vi "Gamepad MicroDrive Control with limits.vi"() -> ()   [LabVIEW 2012]
uses:
  <vilib>/Utility/miscctls.llb/LVPointTypeDef.ctl
  <vilib>/Utility/file.llb/Read From Spreadsheet File (I64).vi
  <vilib>/Utility/inputDevices.llb/closeJoystick.vi
  <vilib>/Utility/inputDevices.llb/joystickAcquire.vi
  <vilib>/Utility/file.llb/Write To Spreadsheet File (DBL).vi
  <vilib>/Utility/file.llb/Read From Spreadsheet File (DBL).vi
  MicroDrive.dll
panel:
  in  "xf":u16(ring)=3 items=["1 X"=1, "2 A"=2, "3 B"=3, "4 Y"=4, "5 LB"=5, "6 RB"=6, "7 LT"=7, "8 RT"=8, "9 Back"=9]
  in  "zf":u16(ring)=6 items=["1 X"=1, "2 A"=2, "3 B"=3, "4 Y"=4, "5 LB"=5, "6 RB"=6, "7 LT"=7, "8 RT"=8, "9 Back"=9]
  in  "Slide 2":cluster{u32, u32, u32}(slide)={0, 1, 5} scale=0.0..7.0
  in  "Invert 2":bool=TRUE
  out "z top":bool
  out "M3 encoder at position":dbl=5.0 step=0.1 format="%_6g"
  in  "M3 low limit":dbl=-10.0 step=0.1 format="%_6g"
  in  "M3 high limit":dbl=10.0 step=0.1 format="%_6g"
  in  "Reset Z":bool
  out "E3 encoder":dbl=5.0 step=0.1 format="%_6g"
  in  "M3 velocity":dbl=1.0 min=0.01905 max=4.0 format="%.3f"
  in  "M3 distance":dbl=1.0 format="%.5f"
  in  "z-down":bool
  in  "z-up":bool
  in  "readWhileMoving":bool=TRUE
  in  "loadLimits":bool
  in  "saveLimits":bool
  in  "roiLoad":bool
  in  "roiSave":bool
  in  "roiRename":bool
  in  "roiName":string
  in  "roiDeleteAll":bool
  out "M2 encoder at position":dbl=5.0 step=0.1 format="%_6g"
  out "M1 encoder at position":dbl=5.0 step=0.1 format="%_6g"
  in  "M2 distance":dbl=1.0 format="%.5f"
  in  "M1 distance":dbl=1.0 format="%.5f"
  out "E2 encoder":dbl=5.0 step=0.1 format="%_6g"
  out "E1 encoder":dbl=5.0 step=0.1 format="%_6g"
  in  "left":bool
  in  "down":bool
  in  "right":bool
  in  "up":bool
  in  "roiMoveTo":bool
  in  "roiDelete":bool
  in  "roiAdd":bool
  in  "ROIs":u16(ring)
  in  "Use software limits":bool=TRUE
  in  "M2 low limit":dbl=-10.0 step=0.1 format="%_6g"
  in  "M2 high limit":dbl=10.0 step=0.1 format="%_6g"
  in  "M1 low limit":dbl=-10.0 step=0.1 format="%_6g"
  in  "M1 high limit":dbl=10.0 step=0.1 format="%_6g"
  in  "closed?":bool
  in  "configure":bool
  in  "device info":bool
  in  "yf":u16(ring)=4 items=["1 X"=1, "2 A"=2, "3 B"=3, "4 Y"=4, "5 LB"=5, "6 RB"=6, "7 LT"=7, "8 RT"=8, "9 Back"=9]
  in  "halt 3":u16(ring)=9 items=["1 X"=1, "2 A"=2, "3 B"=3, "4 Y"=4, "5 LB"=5, "6 RB"=6, "7 LT"=7, "8 RT"=8, "9 Back"=9]
  in  "yr":u16(ring)=2 items=["1 X"=1, "2 A"=2, "3 B"=3, "4 Y"=4, "5 LB"=5, "6 RB"=6, "7 LT"=7, "8 RT"=8, "9 Back"=9]
  in  "zr":u16(ring)=8 items=["1 X"=1, "2 A"=2, "3 B"=3, "4 Y"=4, "5 LB"=5, "6 RB"=6, "7 LT"=7, "8 RT"=8, "9 Back"=9]
  in  "xr":u16(ring)=1 items=["1 X"=1, "2 A"=2, "3 B"=3, "4 Y"=4, "5 LB"=5, "6 RB"=6, "7 LT"=7, "8 RT"=8, "9 Back"=9]
  out "right":bool
  out "left":bool
  out "top":bool
  in  "halt 2":bool
  out "bottom":bool
  out "Max Velocity One Axis":dbl
  out "Min Velocity":dbl
  in  "Reset Both":bool
  in  "Reset Y":bool
  in  "Reset X":bool
  in  "M2 velocity":dbl=1.0 min=0.01905 max=4.0 format="%.3f"
  in  "M1 velocity":dbl=1.0 min=0.01905 max=4.0 format="%.3f"
  out "Max VelocityTwo Axis":dbl format="%.3f"
  in  "Invert":bool=TRUE
  in  "Invert":bool
  out "z bottom":bool
  # "Current Postion"
  # "Single Step Controls"
  # "Stage-Position List"
  # "Encoders"
  # "Step distance"
  # "mm"
  # "mm"
  # "mm"
  # "mm"
  # "mm"
  # "mm"
  # "mm"
  # "mm"
  # "Step velocity"
  # "mm"
  # "mm"
  # "mm"
  # "Read encoders while moving"
  # "Disable if MicroDrive exhibits irregularities while moving."
  # "mm/s"
  # "mm/s"
  # "Rename"
  # "Reset Encoders"
  # "mm/s"
  # "Step Velocity also sets maximum velocity  achievable with gamepad."
  # "Add/Remove"
  # "Reseting encoders will alter Software Limits and erase ROIs"
  # "Software Limits"
  # "(mm)"
  # "Software limits are based on encoder values as displayed above. CAUTION: stage may stop up to 0.5mm beyond specified limit."
  # "Configuration"
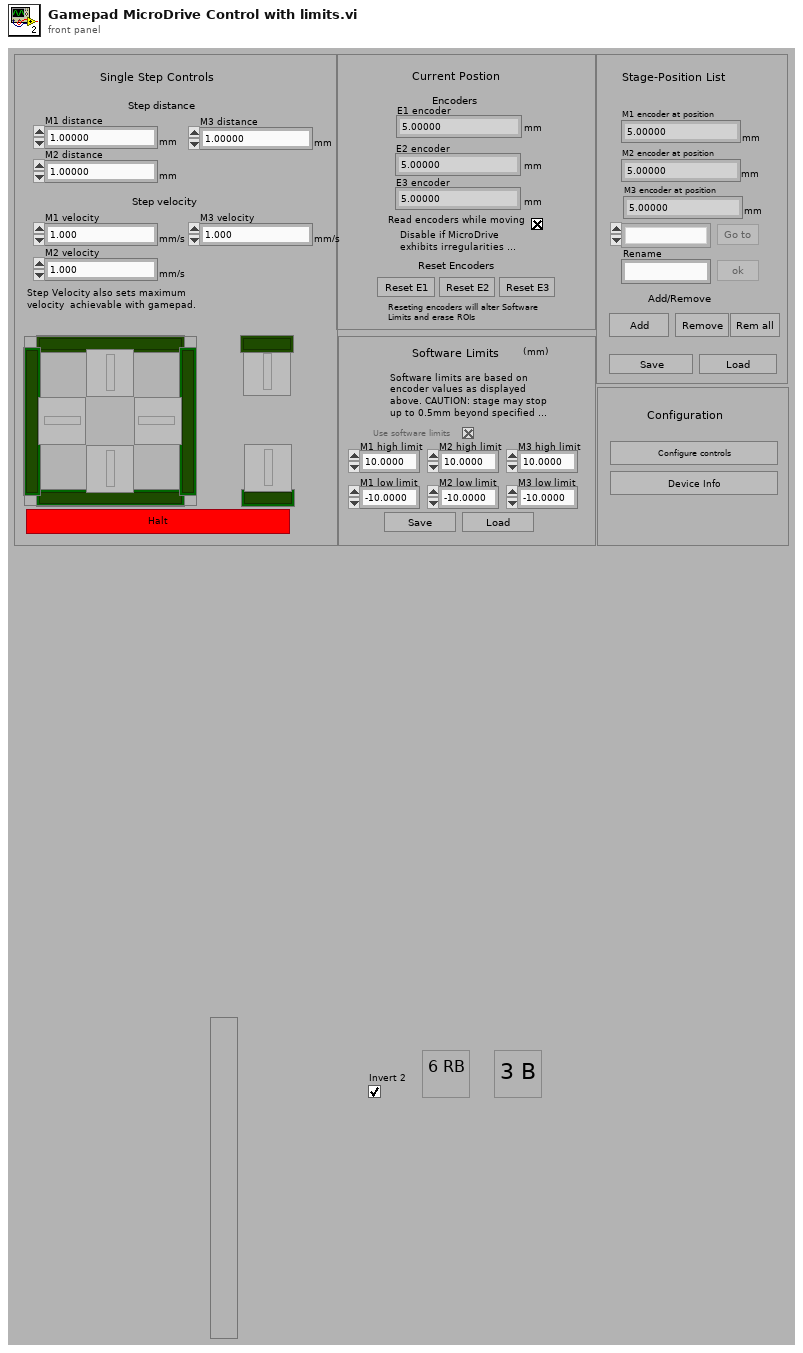
[diagram p1: front panel]
types:
  T1 = enum16{"open", "replace", "create", "open or create", "replace or create", "replace or create with confirmation"}
  T2 = typedef "LVPointTypeDef.ctl" = cluster{"Horizontal":i16, "Vertical":i16}
  T3 = enum8{"Enabled", "Disabled", "Disabled and Grayed Out"}
  T4 = cluster{"Controls":cluster{"Values":cluster{"up":u16, "right":u16}}, "ControlRefs":cluster{"Values":cluster{"up":refnum<vi>, "right":refnum<vi>}}, "Variables":cluster{"Commands":cluster{"up_changed":bool, "right_changed":bool}}}
  T5 = cluster{"Controls":cluster{"Commands":cluster{"right":bool, "left":bool, "up":bool, "down":bool, "z-up":bool, "z-down":bool}, "Values":cluster{"xStep":dbl, "yStep":dbl, "xVelocity":dbl, "yVelocity":dbl, "zStep":dbl, "zVelocity":dbl}}, "ControlRefs":cluster{"Commands":cluster{"right":refnum<vi>, "left":refnum<vi>, "up":refnum<vi>, "down":refnum<vi>, "z-up":refnum<vi>, "z-down":refnum<vi>}, "Values":cluster{"X step":refnum<vi>, "Y step":refnum<vi>, "xVelocity":refnum<vi>, "yVelocity":refnum<vi>, "Z step":refnum<vi>, "zVelocity":refnum<vi>}}}
  T6 = cluster{"Controls":cluster{"Commands":cluster{"Use software limits":bool, "reset X":bool, "reset Y":bool, "reset All":bool, "saveLimits":bool, "loadLimits":bool, "Read encoders while moving":bool, "reset Z":bool}, "Values":cluster{"X high limit":dbl, "X low limit":dbl, "Y high limit":dbl, "Y low limit":dbl, "xEnc":dbl, "yEnc":dbl, "Z high limit":dbl, "Z low limit":dbl, "zEnc":dbl}}, "ControlRefs":cluster{"Commands":cluster{"Use software limits":refnum<vi>, "reset X":refnum<vi>, "reset Y":refnum<vi>, "reset All":refnum<vi>, "saveLimits":refnum<vi>, "loadLimits":refnum<vi>, "Read encoders while moving":refnum<vi>, "reset Z":refnum<vi>}, "Values":cluster{"X high limit":refnum<vi>, "X low limit":refnum<vi>, "Y high limit":refnum<vi>, "Y low limit":refnum<vi>, "xEnc":refnum<vi>, "yEnc":refnum<vi>, "Z high limit":refnum<vi>, "Z low limit":refnum<vi>, "zEnc":refnum<vi>}}, "Variables":cluster{"Commands":cluster{"softLimit_xHigh":bool, "softLimit_xLow":bool, "softLimit_yHigh":bool, "softLimit_yLow":bool, "softLimit_zHigh":bool, "softLimit_zLow ":bool}}}
  T7 = cluster{"Controls":cluster{"Commands":cluster{"roiMoveTo":bool, "roiAdd":bool, "roiDelete":bool, "roiDeleteAll":bool, "rename":bool, "roiSave":bool, "roiLoad":bool}, "Values":cluster{"ROIs":u16, "roiName":string}}, "ControlRefs":cluster{"Commands":cluster{"roiMoveTo":refnum<vi>, "roiAdd":refnum<vi>, "roiDelete":refnum<vi>, "roiDeleteAll":refnum<vi>, "rename":refnum<vi>, "roiSave":refnum<vi>, "roiLoad":refnum<vi>}, "Values":cluster{"ROIs":refnum<vi>, "roiName":refnum<vi>}}, "Variables":cluster{"Values":cluster{"roiText":string[], "ROIs":cluster{"x":dbl, "y":dbl, "z":dbl}[], "roiNumItems":i32}}}
  T8 = cluster{"xr":refnum<vi>, "yr":refnum<vi>, "xf":refnum<vi>, "yf":refnum<vi>, "zr":refnum<vi>, "zf":refnum<vi>, "halt 3":refnum<vi>}
  T9 = cluster{"X axis":i32, "Y axis":i32, "Z axis":i32, "X axis rotation":i32, "Y axis rotation":i32, "Z axis rotation":i32, "U axis":i32, "V axis":i32}
  T10 = cluster{"button 1":bool, "button 2":bool, "button 3":bool, "button 4":bool, "button 5":bool, "button 6":bool, "button 7":bool, "button 8":bool, "button 9":bool, "button 10":bool, "button 11":bool, "button 12":bool, "button 13":bool, "button 14":bool, "button 15":bool, "button 16":bool, "button 17":bool, "button 18":bool, "button 19":bool, "button 20":bool, "button 21":bool, "button 22":bool, "button 23":bool, "button 24":bool, "button 25":bool, "button 26":bool, "button 27":bool, "button 28":bool, "button 29":bool, "button 30":bool, "button 31":bool, "button 32":bool}
  T11 = cluster{"left":bool, "down":bool, "right":bool, "up":bool, "z-up":bool, "z-down":bool, "halt":bool, "button 10":bool}
  T12 = cluster{"y reverse":bool, "y foward":bool, "x reverse":bool, "x foward":bool, "z reverse":bool, "z foward":bool}
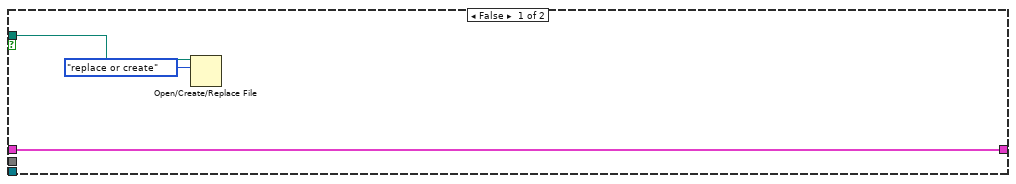
[diagram p2: hidden frame]
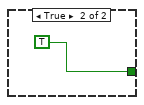
[diagram p4: hidden frame]
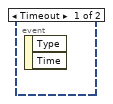
[diagram p8: hidden frame]
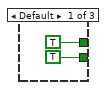
[diagram p13: hidden frame]
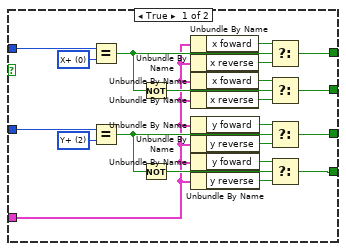
[diagram p15: hidden frame]
diagram:
  n1 = flat-sequence {
    tunnel: [w65] -> w22
    tunnel: [w64] -> w24
    tunnel: [w63] -> w26
    tunnel: [w62] -> w20
    tunnel: [w61] -> w18
    tunnel: w26 -> [w84]
    tunnel: [w84] -> w25
    tunnel: w24 -> [w83]
    tunnel: [w83] -> w23
    tunnel: w22 -> [w82]
    tunnel: [w82] -> w21
    tunnel: w20 -> [w77]
    tunnel: [w75] -> w19
    tunnel: w18 -> [w70]
    tunnel: [w70] -> w17
    tunnel: [w85] -> w10
    tunnel: [w100] -> w8
    tunnel: [w87] -> w6
    tunnel: [w86] -> w4
    tunnel: [w99] -> w2
    tunnel: w17 -> [w99]
    tunnel: w19 -> [w86]
    tunnel: w21 -> [w85]
    tunnel: w23 -> [w95]
    tunnel: w25 -> [w87]
    tunnel: w10 -> [w124]
    tunnel: [w124] -> w9
    tunnel: w8 -> [w123]
    tunnel: [w123] -> w7
    tunnel: w6 -> [w107]
    tunnel: [w106] -> w5
    tunnel: w4 -> [w122]
    tunnel: [w122] -> w3
    tunnel: w2 -> [w121]
    tunnel: [w121] -> w1
    tunnel: w9 -> [w131]
    tunnel: [w125] -> w30
    tunnel: w7 -> [w137]
    tunnel: [w137] -> w29
    tunnel: w5 -> [w136]
    tunnel: [w136] -> w28
    tunnel: w3 -> [w135]
    tunnel: [w135] -> w27
    tunnel: w1 -> [w130]
    tunnel: [w130] -> w16
    tunnel: w30 -> [w145]
    tunnel: [w145] -> w34
    tunnel: w29 -> [w142]
    tunnel: [w142] -> w33
    tunnel: w28 -> [w151]
    tunnel: [w151] -> w32
    tunnel: w27 -> [w150]
    tunnel: [w150] -> w31
    tunnel: w16 -> [w141]
    tunnel: [w140] -> w13
    tunnel: [w204] -> w50
    tunnel: [w207] -> w45
    tunnel: [w206] -> w44
    tunnel: [w205] -> w37
    tunnel: w31 -> [w205]
    tunnel: w32 -> [w206]
    tunnel: w33 -> [w207]
    tunnel: w34 -> [w204]
    tunnel: [w194] -> w14
    tunnel: w13 -> [w194]
    tunnel: [w214] -> w54
    tunnel: [w213] -> w53
    tunnel: w50 -> [w212]
    tunnel: [w212] -> w49
    tunnel: [w211] -> w46
    tunnel: w45 -> [w211]
    tunnel: w44 -> [w210]
    tunnel: [w210] -> w42
    tunnel: [w209] -> w38
    tunnel: w37 -> [w209]
    tunnel: [w208] -> w15
    tunnel: w14 -> [w208]
    tunnel: [w243] -> w60
    tunnel: [w244] -> w58
    tunnel: [w240] -> w56
    tunnel: w54 -> [w244]
    tunnel: w53 -> [w243]
    tunnel: w49 -> [w239]
    tunnel: [w239] -> w47
    tunnel: w46 -> [w237]
    tunnel: [w238] -> w43
    tunnel: w42 -> [w238]
    tunnel: [w237] -> w41
    tunnel: w38 -> [w236]
    tunnel: [w236] -> w35
    tunnel: w15 -> [w235]
    tunnel: [w235] -> w11
    tunnel: w60 -> [w270]
    tunnel: [w270] -> w59
    tunnel: w58 -> [w271]
    tunnel: [w271] -> w57
    tunnel: w56 -> [w269]
    tunnel: [w269] -> w55
    tunnel: [w264] -> w52
    tunnel: [u32 0 ("current button state")] -> w51
    tunnel: [w262] -> w48
    tunnel: w47 -> [w262]
    tunnel: w43 -> [w260]
    tunnel: w41 -> [w261]
    tunnel: [w261] -> w40
    tunnel: [w260] -> w39
    tunnel: [w259] -> w36
    tunnel: w35 -> [w259]
    tunnel: [w258] -> w12
    tunnel: w11 -> [w258]
    tunnel: w55 -> [w279]
    tunnel: w57 -> [w281]
    tunnel: w59 -> [w280]
    tunnel: w52 -> [w278]
    tunnel: w51 -> [w277]
    tunnel: w48 -> [w276]
    tunnel: w40 -> [w275]
    tunnel: w39 -> [w274]
    tunnel: w36 -> [w273]
    tunnel: w12 -> [w272]
    frame #0 {
      w61 = T4 {"Controls"={"Values"={"up"=2, "right"=0}}, "ControlRefs"={"Values"={"up"=refnum, "right"=refnum}}, "Variables"={"Commands"={"up_changed"=FALSE, "right_changed"=FALSE}}}  # Configuration
      w62 = T5 {"Controls"={"Commands"={"right"=FALSE, "left"=FALSE, "up"=FALSE, "down"=FALSE, "z-up"=FALSE, "z-down"=FALSE}, "Values"={"xStep"=1.0, "yStep"=1.0, "xVelocity"=1.0, "yVelocity"=1.0, "zStep"=1.0, "zVelocity"=1.0}}, "ControlRefs"={"Commands"={"right"=refnum, "left"=refnum, "up"=refnum, "down"=refnum, "z-up"=refnum, "z-down"=refnum}, "Values"={"X step"=refnum, "Y step"=refnum, "xVelocity"=refnum, "yVelocity"=refnum, "Z step"=refnum, "zVelocity"=refnum}}}  # Motion
      w63 = T6 {"Controls"={"Commands"={"Use software limits"=FALSE, "reset X"=FALSE, "reset Y"=FALSE, "reset All"=FALSE, "saveLimits"=FALSE, "loadLimits"=FALSE, "Read encoders while moving"=FALSE, "reset Z"=FALSE}, "Values"={"X high limit"=100.0, "X low limit"=-100.0, "Y high limit"=100.0, "Y low limit"=-100.0, "xEnc"=0.0, "yEnc"=0.0, "Z high limit"=100.0, "Z low limit"=-100.0, "zEnc"=0.0}}, "ControlRefs"={"Commands"={"Use software limits"=refnum, "reset X"=refnum, "reset Y"=refnum, "reset All"=refnum, "saveLimits"=refnum, "loadLimits"=refnum, "Read encoders while moving"=refnum, "reset Z"=refnum}, "Values"={"X high limit"=refnum, "X low limit"=refnum, "Y high limit"=refnum, "Y low limit"=refnum, "xEnc"=refnum, "yEnc"=refnum, "Z high limit"=refnum, "Z low limit"=refnum, "zEnc"=refnum}}, "Variables"={"Commands"={"softLimit_xHigh"=FALSE, "softLimit_xLow"=FALSE, "softLimit_yHigh"=FALSE, "softLimit_yLow"=FALSE, "softLimit_zHigh"=FALSE, "softLimit_zLow "=FALSE}}}  # Encoder
      w64 = T7 {"Controls"={"Commands"={"roiMoveTo"=FALSE, "roiAdd"=FALSE, "roiDelete"=FALSE, "roiDeleteAll"=FALSE, "rename"=FALSE, "roiSave"=FALSE, "roiLoad"=FALSE}, "Values"={"ROIs"=0, "roiName"=""}}, "ControlRefs"={"Commands"={"roiMoveTo"=refnum, "roiAdd"=refnum, "roiDelete"=refnum, "roiDeleteAll"=refnum, "rename"=refnum, "roiSave"=refnum, "roiLoad"=refnum}, "Values"={"ROIs"=refnum, "roiName"=refnum}}, "Variables"={"Values"={"roiText"=[], "ROIs"=[], "roiNumItems"=0}}}  # ROIs
      w65 = T8 {"xr"=refnum, "yr"=refnum, "xf"=refnum, "yf"=refnum, "zr"=refnum, "zf"=refnum, "halt 3"=refnum}  # output cluster
    }
    frame #1 {
      n2 = control-ref of="right"() -> (w74:refnum<vi>)
      n3 = control-ref of="left"() -> (w73:refnum<vi>)
      n4 = control-ref of="up"() -> (w72:refnum<vi>)
      n5 = control-ref of="down"() -> (w71:refnum<vi>)
      n6 = control-ref of="z-up"() -> (w69:refnum<vi>)
      n7 = control-ref of="z-down"() -> (w68:refnum<vi>)
      n8 = control-ref of="M1 distance"() -> (w78:refnum<vi>)
      n9 = control-ref of="M2 distance"() -> (w79:refnum<vi>)
      n10 = control-ref of="M1 velocity"() -> (w80:refnum<vi>)
      n11 = control-ref of="M2 velocity"() -> (w81:refnum<vi>)
      n12 = control-ref of="M3 distance"() -> (w67:refnum<vi>)
      n13 = control-ref of="M3 velocity"() -> (w66:refnum<vi>)
      n14 = Bundle By Name(cluster=w77, "ControlRefs.Values.X step"=w78, "ControlRefs.Values.Y step"=w79, "ControlRefs.Values.xVelocity"=w80, "ControlRefs.Values.yVelocity"=w81, "ControlRefs.Values.Z step"=w67, "ControlRefs.Values.zVelocity"=w66) -> (w76:T5)
      n15 = Bundle By Name(cluster=w76, "ControlRefs.Commands.right"=w74, "ControlRefs.Commands.left"=w73, "ControlRefs.Commands.up"=w72, "ControlRefs.Commands.down"=w71, "ControlRefs.Commands.z-up"=w69, "ControlRefs.Commands.z-down"=w68) -> (w75:T5)
    }
    frame #2 {
      n16 = control-ref of="roiName"() -> (w90:refnum<vi>)
      n17 = control-ref of="roiMoveTo"() -> (w98:refnum<vi>)
      n18 = control-ref of="roiAdd"() -> (w97:refnum<vi>)
      n19 = control-ref of="roiDelete"() -> (w96:refnum<vi>)
      n20 = control-ref of="roiDeleteAll"() -> (w92:refnum<vi>)
      n21 = control-ref of="roiRename"() -> (w91:refnum<vi>)
      n22 = control-ref of="roiSave"() -> (w89:refnum<vi>)
      n23 = control-ref of="roiLoad"() -> (w88:refnum<vi>)
      n24 = control-ref of="ROIs"() -> (w93:refnum<vi>)
      n25 = Bundle By Name(cluster=w95, "ControlRefs.Values.ROIs"=w93, "ControlRefs.Values.roiName"=w90) -> (w94:T7)
      n26 = Bundle By Name(cluster=w94, "ControlRefs.Commands.roiMoveTo"=w98, "ControlRefs.Commands.roiAdd"=w97, "ControlRefs.Commands.roiDelete"=w96, "ControlRefs.Commands.roiDeleteAll"=w92, "ControlRefs.Commands.rename"=w91, "ControlRefs.Commands.roiSave"=w89, "ControlRefs.Commands.roiLoad"=w88) -> (w100:T7)
    }
    frame #3 {
      n27 = control-ref of="Use software limits"() -> (w108:refnum<vi>)
      n28 = control-ref of="Reset X"() -> (w114:refnum<vi>)
      n29 = control-ref of="Reset Y"() -> (w115:refnum<vi>)
      n30 = control-ref of="Reset Both"() -> (w116:refnum<vi>)
      n31 = control-ref of="saveLimits"() -> (w119:refnum<vi>)
      n32 = control-ref of="loadLimits"() -> (w120:refnum<vi>)
      n33 = control-ref of="readWhileMoving"() -> (w105:refnum<vi>)
      n34 = control-ref of="Reset Z"() -> (w104:refnum<vi>)
      n35 = Bundle By Name(cluster=w107, "ControlRefs.Commands.Use software limits"=w108, "ControlRefs.Commands.reset X"=w114, "ControlRefs.Commands.reset Y"=w115, "ControlRefs.Commands.reset All"=w116, "ControlRefs.Commands.saveLimits"=w119, "ControlRefs.Commands.loadLimits"=w120, "ControlRefs.Commands.Read encoders while moving"=w105, "ControlRefs.Commands.reset Z"=w104) -> (w113:T6)
      n36 = control-ref of="M1 high limit"() -> (w109:refnum<vi>)
      n37 = control-ref of="M1 low limit"() -> (w110:refnum<vi>)
      n38 = control-ref of="M2 high limit"() -> (w111:refnum<vi>)
      n39 = control-ref of="M2 low limit"() -> (w112:refnum<vi>)
      n40 = control-ref of="E1 encoder"() -> (w117:refnum<vi>)
      n41 = control-ref of="E2 encoder"() -> (w118:refnum<vi>)
      n42 = control-ref of="M3 high limit"() -> (w102:refnum<vi>)
      n43 = control-ref of="M3 low limit"() -> (w101:refnum<vi>)
      n44 = control-ref of="E3 encoder"() -> (w103:refnum<vi>)
      n45 = Bundle By Name(cluster=w113, "ControlRefs.Values.X high limit"=w109, "ControlRefs.Values.X low limit"=w110, "ControlRefs.Values.Y high limit"=w111, "ControlRefs.Values.Y low limit"=w112, "ControlRefs.Values.xEnc"=w117, "ControlRefs.Values.yEnc"=w118, "ControlRefs.Values.Z high limit"=w102, "ControlRefs.Values.Z low limit"=w101, "ControlRefs.Values.zEnc"=w103) -> (w106:T6)
    }
    frame #4 {
      n46 = control-ref of="zr"() -> (w126:refnum<vi>)
      n47 = control-ref of="halt 3"() -> (w129:refnum<vi>)
      n48 = control-ref of="xf"() -> (w128:refnum<vi>)
      n49 = control-ref of="zf"() -> (w127:refnum<vi>)
      n50 = control-ref of="xr"() -> (w134:refnum<vi>)
      n51 = control-ref of="yr"() -> (w133:refnum<vi>)
      n52 = control-ref of="yf"() -> (w132:refnum<vi>)
      n53 = Bundle(cluster=w131, "xr"=w134, "yr"=w133, "xf"=w128, "yf"=w132, "zr"=w127, "zf"=w126, "halt 3"=w129) -> (w125:T8)
    }
    frame #5 {
      n54 = control-ref of="This Application"() -> (w149:refnum<vi>)
      n55 = property class="App"(reference=w149) -> ("App.Dir"=w144:path)  [unwired: 1 in, 2 out]
      n56 = control-ref of="Slide 2"() -> (w138:refnum<vi>)
      n57 = Build Path(base path=w144, name or relative path="config.txt") -> (appended path=w147:path)
      n58 = Cluster To Array(cluster=w145) -> (array=w146:refnum<vi>[])
      n59 = call <vilib>:"Check if File or Folder Exists.vi"("path"=w147) -> ("file or folder exists?"=w139:bool, "dup path"=w143:path)  [unwired: 1 in, 8 out]
      n60 = case shown="True" w139 {
        tunnel: w138 -> [_ w168]
        tunnel: w146 -> [_ w167]
        tunnel: w143 -> [w154 w166]
        tunnel: w141 -> [w152 w156]
        tunnel: [w152 w155] -> w140
        frame False {
          n61 = Open/Create/Replace File(file path (use dialog)=w154, operation (0:open)=T1."replace or create") -> ()  [unwired: 1 in, 6 out]
        }
        frame True {
          n62 = Read from Text File(file (use dialog)=w166) -> (text=w165:string)  [unwired: 1 in, 5 out]
          n63 = String To Path(string=w165) -> (path=w164:path)
          n64 = call <vilib>:"Check if File or Folder Exists.vi"("path"=w164) -> ("file or folder exists?"=w162:bool, "dup path"=w158:path)  [unwired: 1 in, 8 out]
          n65 = Not A Number/Path/Refnum?(number/path/refnum=w158) -> (NaN/Path/Refnum?=w161:bool)
          n66 = Empty String/Path?(string/path=w158) -> (empty?=w159:bool)
          n67 = Not(x=w161) -> (.not. x?=w160:bool)
          n68 = Not(x=w159) -> (.not. x?=w157:bool)
          n69 = Compound Arithmetic op=AND(w160, w162, w157) -> (w163:bool)
          n70 = case shown="True" w163 {
            tunnel: w167 -> [_ w188]
            tunnel: w168 -> [_ w189]
            tunnel: w158 -> [_ w187]
            tunnel: w156 -> [w169 w186]
            tunnel: [w169 w185] -> w155
            frame False {
            }
            frame True {
              n71 = call-poly <vilib>:"Read From Spreadsheet File.vi"("transpose (no:F)"=TRUE ("transpose? (no:F)"), "file path (dialog if empty)"=w187) -> ("first row"=w190:i64[])  [unwired: 2 in, 7 out]
              n72 = Array Size(array=w188) -> (size(s)=w184:i32)
              n73 = Split 1D Array(array=w190, index=w184) -> (first subarray=w181:i64[], second subarray=w183:i64[])
              n74 = Index Array(array=w183) -> (element #1=w175:i64, element #2=w176:i64, element #3=w170:i64, element #4=w171:i64, element #5=w172:i64, element #6=w173:i64, element #7=w174:i64)  [unwired: 7 in]
              n75 = Bundle(w176, w175, w170) -> (w182:cluster{i64, i64, i64})  [unwired: 1 out]
              n76 = property class="Slide (strict)"(reference=w189, "Value"=w182) -> ()  [unwired: 1 in, 2 out]
              n77 = Bundle By Name(cluster=w186, "Controls.Values.up"=w173, "Controls.Values.right"=w174) -> (w185:T4)
              n78 = control-ref of="Invert"() -> (w178:refnum<vi>)
              n79 = control-ref of="Invert"() -> (w177:refnum<vi>)
              n80 = Greater Than 0?(x=w171) -> (x > 0?=w180:bool)
              n81 = Greater Than 0?(x=w172) -> (x > 0?=w179:bool)
              n82 = property class="Bool (strict)"(reference=w178, "Value"=w180) -> ()  [unwired: 1 in, 2 out]
              n83 = property class="Bool (strict)"(reference=w177, "Value"=w179) -> ()  [unwired: 1 in, 2 out]
              n84 = for {
                tunnel: w188 -> [w193] mode=indexing
                tunnel: w181 -> [w192] mode=indexing
                n85 = property class="Ring (strict)"(reference=w193, "Value"=w192) -> ()  [unwired: 1 in, 2 out]
              }
            }
          }
        }
      }
    }
    frame #6 {
      w195 = u16 0  # Value
      w196 = string[] []  # Strings
      w200 = TRUE ("Front Panel Window:Closeable")
      w201 = FALSE ("Front Panel Window:Title Bar Visible")
      n86 = Unbundle By Name(w207) -> ("ControlRefs.Values.ROIs"=w197:refnum<vi>)
      n87 = control-ref of="This VI"() -> (w203:refnum<vi>)
      n88 = control-ref of="Pane"() -> (w198:refnum<vi>)
      n89 = property class="Ring (strict)"(reference=w197, "Strings []"=w196, "Value"=w195) -> ()  [unwired: 1 in, 2 out]
      n90 = property class="VI"(reference=w203, "Front Panel.Title"="MicroDrive Gamepad" ("Front Panel Window:Title"), "Front Panel.TitleBarVis"=w200, "TB.Visible"=w201, "Front Panel.ShowMenuBar"=w201, "Front Panel.Closeable"=w200) -> ()  [unwired: 1 in, 2 out]
      n91 = property class="Pane"(reference=w198, "Origin"=T2 {"Horizontal"=0, "Vertical"=0}) -> ()  [unwired: 1 in, 2 out]
    }
    frame #7 {
      n92 = while {
        tunnel: [w220] -> w213
        tunnel: [w215] -> w214
        stop <- w219 stop-if-true
        n93 = flat-sequence {
          tunnel: [w223] -> w222
          tunnel: [w224] -> w221
          tunnel: [w223] -> w218
          tunnel: w222 -> [w228]
          tunnel: [w227] -> w220
          tunnel: w221 -> [w227]
          tunnel: [w226] -> w215
          tunnel: w218 -> [w226]
          tunnel: [w225] -> w217
          frame #0 {
            n94 = call "init joystick.vi"() -> ("device ID"=w224:refnum<k1>, "Joystick found"=w223:bool)  [unwired: 2 out]
          }
          frame #1 {
            n95 = case shown="False" w228 {
              tunnel: [w229 TRUE ("T button?")] -> w225
              frame False {
                n96 = Two Button Dialog(message="Press start (button 10)\n on your Gamepad \n(while pressing 'Ok')\nfor it to be initialized. ", 1:"Cancel Program" ("F button name (\"Cancel\")"), 2:"Ok" ("T button name (\"OK\")")) -> (T button?=w229:bool)
              }
              frame True {
              }
            }
          }
        }
        n97 = Not(x=w217) -> (.not. x?=w216:bool)
        n98 = Or(x=w216, y=w215) -> (x .or. y?=w219:bool)
      }
    }
    frame #8 {
      n99 = dll-call lib="C:/Users/Labview/Desktop/SRR/MicroDrive_x64/Labview Examples/MicroDrive.dll" fn="MCL_InitHandleOrGetExisting"() -> ("return type"=w241:i32)  [unwired: 3 in, 2 out]
      n100 = Less Or Equal To 0?(x=w241) -> (x <= 0?=w242:bool)
      n101 = case shown="True" w242 {
        tunnel: w241 -> [w245 w248]
        tunnel: [w245 w247] -> w240
        tunnel: "Retry" ("T button name (\"OK\")") -> [_ w246]
        frame False {
        }
        frame True {
          n102 = while {
            tunnel: w248 -> [w254]
            tunnel: [w252] -> w247
            tunnel: w246 -> [w249]
            stop <- w251 continue-if-true
            n103 = Two Button Dialog(message="Failed to load MicroDrive!\nRetry?", 2:w249) -> (T button?=w250:bool)  [unwired: 1 out]
            n104 = case shown="True" w250 {
              tunnel: w254 -> [w256 _]
              tunnel: [w256 w257] -> w252
              frame False {
              }
              frame True {
                n105 = dll-call lib="C:/Users/Labview/Desktop/SRR/MicroDrive_x64/Labview Examples/MicroDrive.dll" fn="MCL_InitHandleOrGetExisting"() -> ("return type"=w257:i32)  [unwired: 3 in, 2 out]
              }
            }
            n106 = Less Or Equal To 0?(x=w252) -> (x <= 0?=w253:bool)
            n107 = And(x=w250, y=w253) -> (x .and. y?=w251:bool)
          }
        }
      }
    }
    frame #9 {
      n108 = call "device in.vi"("handle"=w269) -> ("Out"=w264:string, "minVelocity"=→"Min Velocity":dbl, "maxVelocityTwoAxis"=→"Max VelocityTwo Axis":dbl, "maxVelocity"=→"Max Velocity One Axis":dbl)  [unwired: 15 out]
      n109 = local write "closed?"(FALSE ("closed?")) -> ()
    }
    frame #10 {
      n110 = case shown="True" w281 {
        tunnel: w280 -> [_ w293]
        tunnel: w279 -> [_ w290]
        tunnel: w278 -> [_ w289]
        tunnel: w277 -> [_ w287]
        tunnel: w276 -> [_ w286]
        tunnel: w275 -> [_ w285]
        tunnel: w274 -> [_ w284]
        tunnel: w273 -> [_ w283]
        tunnel: w272 -> [_ w282]
        frame False {
        }
        frame True {
          n111 = while {
            tunnel: w293 -> [w537]
            tunnel: [w536] -> w292
            tunnel: [w535] -> w291
            tunnel: w290 -> [w534]
            shift-right: [w527] -> _
            shift-left: w287 -> [w526]
            tunnel: w289 -> [w525]
            tunnel: w286 -> [w517]
            shift-right: [w479] -> _
            shift-left: w285 -> [w495]
            shift-right: [w478] -> _
            shift-left: w284 -> [w494]
            tunnel: w283 -> [w477]
            shift-right: [w401] -> _
            shift-left: w282 -> [w417]
            stop <- w524 stop-if-true
            n112 = flat-sequence {
              tunnel: w477 -> [w546]
              tunnel: w494 -> [w547]
              tunnel: w495 -> [w548]
              tunnel: w517 -> [w549]
              tunnel: w537 -> [w550]
              tunnel: w534 -> [w551]
              tunnel: w526 -> [w552]
              tunnel: w525 -> [w553]
              tunnel: [w553] -> w425
              tunnel: [w552] -> w424
              tunnel: [w551] -> w423
              tunnel: [w550] -> w422
              tunnel: [w549] -> w421
              tunnel: [w548] -> w420
              tunnel: [w547] -> w419
              tunnel: [w545] -> w418
              tunnel: w417 -> [w540]
              tunnel: [w540] -> w416
              tunnel: [w577] -> w382
              tunnel: [w576] -> w380
              tunnel: [w575] -> w378
              tunnel: [w574] -> w376
              tunnel: [w573] -> w374
              tunnel: [w572] -> w372
              tunnel: [w559] -> w370
              tunnel: [w571] -> w368
              tunnel: [w570] -> w366
              tunnel: w416 -> [w570]
              tunnel: w418 -> [w563]
              tunnel: w419 -> [w559]
              tunnel: w420 -> [w566]
              tunnel: w421 -> [w573]
              tunnel: w422 -> [w574]
              tunnel: w423 -> [w575]
              tunnel: w424 -> [w576]
              tunnel: w425 -> [w577]
              tunnel: w382 -> [w602]
              tunnel: [w602] -> w381
              tunnel: w380 -> [w601]
              tunnel: [w601] -> w379
              tunnel: w378 -> [w600]
              tunnel: [w600] -> w377
              tunnel: w376 -> [w599]
              tunnel: [w599] -> w375
              tunnel: w374 -> [w598]
              tunnel: [w598] -> w373
              tunnel: w372 -> [w597]
              tunnel: [w597] -> w371
              tunnel: w370 -> [w585]
              tunnel: [w584] -> w369
              tunnel: w368 -> [w596]
              tunnel: [w596] -> w367
              tunnel: w366 -> [w595]
              tunnel: [w595] -> w365
              tunnel: w381 -> [w615]
              tunnel: [w615] -> w315
              tunnel: w379 -> [w614]
              tunnel: [w614] -> w313
              tunnel: w377 -> [w613]
              tunnel: [w613] -> w311
              tunnel: w375 -> [w612]
              tunnel: [w612] -> w309
              tunnel: w373 -> [w611]
              tunnel: [w611] -> w307
              tunnel: w371 -> [w610]
              tunnel: [w610] -> w305
              tunnel: w369 -> [w609]
              tunnel: [w609] -> w303
              tunnel: w367 -> [w608]
              tunnel: [w607] -> w301
              tunnel: w365 -> [w604]
              tunnel: [w604] -> w299
              tunnel: w315 -> [w634]
              tunnel: [w634] -> w314
              tunnel: w313 -> [w633]
              tunnel: [w633] -> w312
              tunnel: w311 -> [w632]
              tunnel: [w632] -> w310
              tunnel: w309 -> [w631]
              tunnel: [w631] -> w308
              tunnel: w307 -> [w627]
              tunnel: [w627] -> w306
              tunnel: w305 -> [w628]
              tunnel: [w628] -> w304
              tunnel: w303 -> [w622]
              tunnel: [w616] -> w302
              tunnel: w301 -> [w630]
              tunnel: [w630] -> w300
              tunnel: w299 -> [w629]
              tunnel: [w629] -> w298
              tunnel: [w649] -> w523
              tunnel: [w648] -> w521
              tunnel: [w647] -> w519
              tunnel: [w644] -> w515
              tunnel: w314 -> [w645]
              tunnel: w312 -> [w649]
              tunnel: w310 -> [w648]
              tunnel: w308 -> [w647]
              tunnel: w306 -> [w644]
              tunnel: [w643] -> w493
              tunnel: w304 -> [w643]
              tunnel: [w642] -> w492
              tunnel: w302 -> [w642]
              tunnel: [w641] -> w475
              tunnel: w300 -> [w641]
              tunnel: w298 -> [w640]
              tunnel: [w640] -> w414
              tunnel: w523 -> [w660]
              tunnel: [w660] -> w522
              tunnel: w521 -> [w651]
              tunnel: [w651] -> w520
              tunnel: w519 -> [w658]
              tunnel: [w658] -> w518
              tunnel: [w657] -> w516
              tunnel: w515 -> [w657]
              tunnel: w493 -> [w656]
              tunnel: w492 -> [w655]
              tunnel: [w656] -> w491
              tunnel: [w655] -> w490
              tunnel: [w654] -> w476
              tunnel: w475 -> [w654]
              tunnel: [w652] -> w415
              tunnel: w414 -> [w653]
              tunnel: [w685] -> w451
              tunnel: [w673] -> w449
              tunnel: [w684] -> w447
              tunnel: w522 -> [w684]
              tunnel: w520 -> [w673]
              tunnel: w518 -> [w685]
              tunnel: w516 -> [w683]
              tunnel: [w683] -> w445
              tunnel: [w682] -> w443
              tunnel: w491 -> [w682]
              tunnel: [w680] -> w441
              tunnel: w490 -> [w681]
              tunnel: w476 -> [w679]
              tunnel: [w679] -> w439
              tunnel: w415 -> [w678]
              tunnel: [w678] -> w412
              tunnel: w451 -> [w719]
              tunnel: [w719] -> w450
              tunnel: w449 -> [w718]
              tunnel: [w718] -> w448
              tunnel: w447 -> [w717]
              tunnel: [w717] -> w446
              tunnel: w445 -> [w716]
              tunnel: [w716] -> w444
              tunnel: w443 -> [w715]
              tunnel: [w715] -> w442
              tunnel: w441 -> [w693]
              tunnel: [w702] -> w440
              tunnel: w439 -> [w714]
              tunnel: [w714] -> w438
              tunnel: [w698] -> w413
              tunnel: w412 -> [w698]
              tunnel: [w729] -> w400
              tunnel: [w728] -> w399
              tunnel: [w727] -> w398
              tunnel: [w726] -> w397
              tunnel: [w720] -> w396
              tunnel: [w725] -> w395
              tunnel: [w724] -> w394
              tunnel: [w723] -> w393
              tunnel: [w722] -> w392
              tunnel: [w721] -> w391
              tunnel: w413 -> [w721]
              tunnel: w438 -> [w722]
              tunnel: w440 -> [w723]
              tunnel: w442 -> [w724]
              tunnel: w444 -> [w726]
              tunnel: w446 -> [w727]
              tunnel: w448 -> [w728]
              tunnel: w450 -> [w729]
              tunnel: w400 -> [w740]
              tunnel: [w740] -> w514
              tunnel: w399 -> [w739]
              tunnel: [w739] -> w512
              tunnel: w398 -> [w736]
              tunnel: [w736] -> w510
              tunnel: w397 -> [w737]
              tunnel: w396 -> [w735]
              tunnel: [w730] -> w508
              tunnel: w395 -> [w738]
              tunnel: [w738] -> w506
              tunnel: w394 -> [w734]
              tunnel: w393 -> [w733]
              tunnel: [w734] -> w488
              tunnel: [w733] -> w486
              tunnel: w392 -> [w732]
              tunnel: [w732] -> w472
              tunnel: w391 -> [w731]
              tunnel: [w731] -> w411
              tunnel: w514 -> [w750]
              tunnel: [w750] -> w513
              tunnel: w512 -> [w749]
              tunnel: [w749] -> w511
              tunnel: w510 -> [w748]
              tunnel: [w748] -> w509
              tunnel: w508 -> [w745]
              tunnel: [w745] -> w507
              tunnel: w506 -> [w747]
              tunnel: [w747] -> w505
              tunnel: [w744] -> w489
              tunnel: w488 -> [w744]
              tunnel: [w743] -> w487
              tunnel: w486 -> [w743]
              tunnel: [w742] -> w473
              tunnel: w472 -> [w742]
              tunnel: w411 -> [w741]
              tunnel: [w741] -> w409
              tunnel: [w795] -> w533
              tunnel: [w798] -> w532
              tunnel: [w797] -> w531
              tunnel: [w796] -> w530
              tunnel: w513 -> [w795]
              tunnel: w511 -> [w798]
              tunnel: [w771] -> w529
              tunnel: w509 -> [w770]
              tunnel: [w770] -> w528
              tunnel: w507 -> [w771]
              tunnel: w505 -> [w772]
              tunnel: w489 -> [w769]
              tunnel: w487 -> [w768]
              tunnel: [w769] -> w485
              tunnel: [w768] -> w484
              tunnel: [w767] -> w474
              tunnel: w473 -> [w767]
              tunnel: [w766] -> w410
              tunnel: w409 -> [w766]
              tunnel: [w764] -> w296
              tunnel: [w818] -> w504
              tunnel: [w820] -> w502
              tunnel: [w816] -> w500
              tunnel: w528 -> [w816]
              tunnel: w529 -> [w799]
              tunnel: w530 -> [w813]
              tunnel: w531 -> [w819]
              tunnel: w532 -> [w820]
              tunnel: w533 -> [w818]
              tunnel: [w812] -> w498
              tunnel: [w804] -> w497
              tunnel: [w802] -> w496
              tunnel: w485 -> [w811]
              tunnel: w484 -> [w810]
              tunnel: [w811] -> w482
              tunnel: [w810] -> w480
              tunnel: w474 -> [w806]
              tunnel: [w806] -> w470
              tunnel: w410 -> [w807]
              tunnel: [w807] -> w407
              tunnel: [w803] -> w297
              tunnel: w296 -> [w801]
              tunnel: w504 -> [w836]
              tunnel: [w836] -> w503
              tunnel: w502 -> [w837]
              tunnel: [w837] -> w501
              tunnel: w500 -> [w843]
              tunnel: [w843] -> w499
              tunnel: w498 -> [w821]
              tunnel: w497 -> [w835]
              tunnel: w496 -> [w834]
              tunnel: [w833] -> w483
              tunnel: w482 -> [w833]
              tunnel: [w832] -> w481
              tunnel: w480 -> [w832]
              tunnel: [w829] -> w471
              tunnel: w470 -> [w829]
              tunnel: [w828] -> w408
              tunnel: w407 -> [w828]
              tunnel: w297 -> [w825]
              tunnel: w503 -> [w878]
              tunnel: w501 -> [w871]
              tunnel: w499 -> [w870]
              tunnel: [w878] -> w390
              tunnel: [w871] -> w389
              tunnel: [w870] -> w388
              tunnel: w483 -> [w869]
              tunnel: w481 -> [w867]
              tunnel: [w869] -> w387
              tunnel: [w867] -> w386
              tunnel: w471 -> [w868]
              tunnel: [w868] -> w385
              tunnel: w408 -> [w866]
              tunnel: [w866] -> w384
              tunnel: [w864] -> w383
              tunnel: [w899] -> w457
              tunnel: [w879] -> w456
              tunnel: [w898] -> w455
              tunnel: [w897] -> w454
              tunnel: [w896] -> w453
              tunnel: [w895] -> w452
              tunnel: [w889] -> w406
              tunnel: w383 -> [w885]
              tunnel: w384 -> [w889]
              tunnel: w385 -> [w895]
              tunnel: w386 -> [w896]
              tunnel: w387 -> [w897]
              tunnel: w388 -> [w898]
              tunnel: w389 -> [w879]
              tunnel: w390 -> [w899]
              tunnel: w457 -> [w961]
              tunnel: [w961] -> w437
              tunnel: w456 -> [w960]
              tunnel: [w960] -> w435
              tunnel: w455 -> [w959]
              tunnel: [w959] -> w433
              tunnel: w454 -> [w956]
              tunnel: [w956] -> w431
              tunnel: w453 -> [w958]
              tunnel: [w958] -> w429
              tunnel: w452 -> [w957]
              tunnel: [w957] -> w427
              tunnel: w406 -> [w949]
              tunnel: [w949] -> w404
              tunnel: w437 -> [w975]
              tunnel: [w975] -> w436
              tunnel: w435 -> [w974]
              tunnel: [w974] -> w434
              tunnel: w433 -> [w973]
              tunnel: [w973] -> w432
              tunnel: w431 -> [w970]
              tunnel: [w970] -> w430
              tunnel: w429 -> [w972]
              tunnel: [w972] -> w428
              tunnel: w427 -> [w971]
              tunnel: [w971] -> w426
              tunnel: [w964] -> w405
              tunnel: w404 -> [w964]
              tunnel: w436 -> [w986]
              tunnel: [w986] -> w364
              tunnel: w434 -> [w985]
              tunnel: [w985] -> w362
              tunnel: w432 -> [w984]
              tunnel: [w984] -> w360
              tunnel: w430 -> [w982]
              tunnel: [w979] -> w358
              tunnel: w428 -> [w978]
              tunnel: [w978] -> w356
              tunnel: w426 -> [w977]
              tunnel: [w977] -> w354
              tunnel: w405 -> [w976]
              tunnel: [w976] -> w352
              tunnel: w364 -> [w1028]
              tunnel: [w1028] -> w363
              tunnel: w362 -> [w1027]
              tunnel: [w1027] -> w361
              tunnel: w360 -> [w1026]
              tunnel: [w1026] -> w359
              tunnel: w358 -> [w1021]
              tunnel: [w1020] -> w357
              tunnel: w356 -> [w1025]
              tunnel: [w1025] -> w355
              tunnel: w354 -> [w1024]
              tunnel: [w1024] -> w353
              tunnel: w352 -> [w1023]
              tunnel: [w1023] -> w351
              tunnel: w363 -> [w1049]
              tunnel: [w1049] -> w469
              tunnel: w361 -> [w1048]
              tunnel: [w1048] -> w467
              tunnel: w359 -> [w1047]
              tunnel: [w1047] -> w465
              tunnel: w357 -> [w1046]
              tunnel: [w1044] -> w463
              tunnel: w355 -> [w1045]
              tunnel: [w1045] -> w461
              tunnel: w353 -> [w1043]
              tunnel: [w1043] -> w459
              tunnel: w351 -> [w1042]
              tunnel: [w1042] -> w402
              tunnel: w469 -> [w1073]
              tunnel: [w1073] -> w468
              tunnel: w467 -> [w1072]
              tunnel: [w1072] -> w466
              tunnel: w465 -> [w1071]
              tunnel: [w1071] -> w464
              tunnel: w463 -> [w1068]
              tunnel: [w1066] -> w462
              tunnel: w461 -> [w1067]
              tunnel: [w1067] -> w460
              tunnel: w459 -> [w1070]
              tunnel: [w1070] -> w458
              tunnel: [w1065] -> w403
              tunnel: w402 -> [w1065]
              tunnel: w468 -> [w1084]
              tunnel: [w1084] -> w350
              tunnel: w466 -> [w1085]
              tunnel: [w1085] -> w349
              tunnel: w464 -> [w1090]
              tunnel: [w1090] -> w348
              tunnel: w462 -> [w1088]
              tunnel: [w1088] -> w347
              tunnel: w460 -> [w1087]
              tunnel: [w1087] -> w346
              tunnel: w458 -> [w1086]
              tunnel: [w1086] -> w345
              tunnel: w403 -> [w1083]
              tunnel: [w1083] -> w344
              tunnel: w350 -> [w1128]
              tunnel: [w1128] -> w343
              tunnel: w349 -> [w1127]
              tunnel: [w1127] -> w342
              tunnel: w348 -> [w1126]
              tunnel: [w1126] -> w341
              tunnel: w347 -> [w1119]
              tunnel: [w1119] -> w340
              tunnel: w346 -> [w1125]
              tunnel: [w1125] -> w339
              tunnel: w345 -> [w1124]
              tunnel: [w1124] -> w338
              tunnel: w344 -> [w1123]
              tunnel: [w1123] -> w337
              tunnel: w343 -> [w1183]
              tunnel: [w1183] -> w336
              tunnel: w342 -> [w1182]
              tunnel: [w1182] -> w335
              tunnel: w341 -> [w1181]
              tunnel: [w1181] -> w334
              tunnel: w340 -> [w1176]
              tunnel: [w1175] -> w333
              tunnel: w339 -> [w1180]
              tunnel: [w1180] -> w332
              tunnel: w338 -> [w1179]
              tunnel: [w1179] -> w331
              tunnel: w337 -> [w1178]
              tunnel: [w1178] -> w330
              tunnel: w336 -> [w1264]
              tunnel: [w1264] -> w329
              tunnel: w335 -> [w1263]
              tunnel: [w1263] -> w327
              tunnel: w334 -> [w1262]
              tunnel: [w1262] -> w325
              tunnel: w333 -> [w1261]
              tunnel: [w1261] -> w323
              tunnel: w332 -> [w1258]
              tunnel: [w1258] -> w321
              tunnel: w331 -> [w1260]
              tunnel: [w1260] -> w319
              tunnel: w330 -> [w1259]
              tunnel: [w1259] -> w317
              tunnel: w329 -> [w1306]
              tunnel: [w1306] -> w328
              tunnel: w327 -> [w1305]
              tunnel: [w1305] -> w326
              tunnel: w325 -> [w1304]
              tunnel: [w1304] -> w324
              tunnel: w323 -> [w1303]
              tunnel: [w1303] -> w322
              tunnel: w321 -> [w1299]
              tunnel: [w1299] -> w320
              tunnel: w319 -> [w1302]
              tunnel: [w1302] -> w318
              tunnel: w317 -> [w1301]
              tunnel: [w1301] -> w316
              tunnel: [w1334] -> w527
              tunnel: [w1335] -> w535
              tunnel: [w1336] -> w536
              tunnel: w328 -> [w1336]
              tunnel: w326 -> [w1335]
              tunnel: w324 -> [w1334]
              tunnel: ["closed?"] -> w524
              tunnel: w322 -> [w1332]
              tunnel: [w1332] -> w479
              tunnel: [w1331] -> w478
              tunnel: w320 -> [w1331]
              tunnel: w318 -> [_]
              tunnel: [w1330] -> w401
              tunnel: w316 -> [w1330]
              frame #0 {
                # "Update control values"
                n113 = Bundle By Name(cluster=w546, "Controls.Commands.right"="right", "Controls.Commands.left"="left", "Controls.Commands.up"="up", "Controls.Commands.down"="down", "Controls.Commands.z-up"="z-up", "Controls.Commands.z-down"="z-down") -> (w545:T5)
              }
              frame #1 {
                # "Update control values"
                n114 = Bundle By Name(cluster=w563, "Controls.Values.xStep"="M1 distance", "Controls.Values.yStep"="M2 distance", "Controls.Values.zStep"="M3 distance") -> (w571:T5)
                n115 = Bundle By Name(cluster=w566, "Controls.Values.ROIs"="ROIs", "Controls.Values.roiName"="roiName") -> (w565:T7)
                n116 = Bundle By Name(cluster=w565, "Controls.Commands.roiMoveTo"="roiMoveTo", "Controls.Commands.roiAdd"="roiAdd", "Controls.Commands.roiDelete"="roiDelete", "Controls.Commands.roiDeleteAll"="roiDeleteAll", "Controls.Commands.rename"="roiRename", "Controls.Commands.roiSave"="roiSave", "Controls.Commands.roiLoad"="roiLoad") -> (w572:T7)
              }
              frame #2 {
                # "Update control values"
                n117 = Bundle By Name(cluster=w585, "Controls.Values.X high limit"="M1 high limit", "Controls.Values.X low limit"="M1 low limit", "Controls.Values.Y high limit"="M2 high limit", "Controls.Values.Y low limit"="M2 low limit", "Controls.Values.Z high limit"="M3 high limit", "Controls.Values.Z low limit"="M3 low limit") -> (w590:T6)
                n118 = Bundle By Name(cluster=w590, "Controls.Commands.reset Z"="Reset Z", "Controls.Commands.Use software limits"="Use software limits", "Controls.Commands.reset X"="Reset X", "Controls.Commands.reset Y"="Reset Y", "Controls.Commands.reset All"="Reset Both", "Controls.Commands.saveLimits"="saveLimits", "Controls.Commands.loadLimits"="loadLimits", "Controls.Commands.Read encoders while moving"="readWhileMoving") -> (w584:T6)
              }
              frame #3 {
                # "Update control values"
                n119 = Bundle By Name(cluster=w608, "Controls.Values.xVelocity"="M1 velocity", "Controls.Values.yVelocity"="M2 velocity", "Controls.Values.zVelocity"="M3 velocity") -> (w607:T5)
              }
              frame #4 {
                # "Don't allow software limits if \"read encoders while moving\" is disabled."
                n120 = Unbundle By Name(w622) -> ("Controls.Commands.Read encoders while moving"=w618:bool)
                n121 = Unbundle By Name(w622) -> ("ControlRefs.Commands.Use software limits"=w621:refnum<vi>, "Controls.Commands.Use software limits"=w624:bool, "Controls.Commands.Read encoders while moving"=w626:bool)
                n122 = Not(x=w626) -> (.not. x?=w625:bool)
                n123 = Compound Arithmetic op=AND(w624, w625) -> (w623:bool)
                n124 = case shown="True" w623 {
                  tunnel: w622 -> [w635 w639]
                  tunnel: [w635 w638] -> w616
                  tunnel: w621 -> [_ w637]
                  frame False {
                  }
                  frame True {
                    w636 = FALSE ("Value")
                    n125 = Bundle By Name(cluster=w639, "Controls.Commands.Use software limits"=w636) -> (w638:T6)
                    n126 = property class="Bool (strict)"(reference=w637, "Value"=w636) -> ()  [unwired: 1 in, 2 out]
                  }
                }
                n127 = Select(t=T3."Enabled" ("Disabled"), s=w618, f=T3."Disabled and Grayed Out" ("Disabled")) -> (s? t:f=w617:T3)
                n128 = property class="Bool (strict)"(reference=w621, "DisabledEnum"=w617) -> ()  [unwired: 1 in, 2 out]
              }
              frame #5 {
                # "Display device info"
                n129 = case shown="True" "device info" {
                  tunnel: w645 -> [_ w650]
                  frame False {
                  }
                  frame True {
                    n130 = One Button Dialog(message=w650) -> ()  [unwired: 2 out]
                  }
                }
              }
              frame #6 {
                # "Configure the Gamepad control stick and buttons."
                n131 = case shown="True" "configure" {
                  tunnel: w658 -> [_ w667]
                  tunnel: w657 -> [_ w666]
                  tunnel: w653 -> [w661 w665]
                  tunnel: [w661 w664] -> w652
                  frame False {
                  }
                  frame True {
                    n132 = control-ref of="Invert"() -> (w669:refnum<vi>)
                    n133 = control-ref of="Invert"() -> (w668:refnum<vi>)
                    n134 = control-ref of="Slide 2"() -> (w663:refnum<vi>)
                    n135 = control-ref of="Invert 2"() -> (w662:refnum<vi>)
                    n136 = call "Configure Gamepad.vi"("invert z"=w662, "Cluster"=w666, "Configuration"=w665, "Slide 2"=w663, "invert y"=w668, "invert x"=w669, "device ID"=w667) -> ("Configuration"=w664:T4)  [unwired: 4 out]
                  }
                }
              }
              frame #7 {
                # "Read the Encoders"
                n137 = Unbundle By Name(w681) -> ("Controls.Commands.reset X"=w677:bool, "Controls.Commands.reset Y"=w676:bool, "Controls.Commands.reset Z"=w675:bool, "Controls.Commands.reset All"=w674:bool)
                n138 = call "read.vi"("handle"=w673, "Reset M1"=w677, "Reset M2"=w676, "Reset M3"=w675, "Reset Encoders"=w674) -> ("M1 pos"=w672:dbl, "M2 pos"=w671:dbl, "M3 pos"=w670:dbl)  [unwired: 8 in]
                "E1 encoder" <- w672
                "E2 encoder" <- w671
                "E3 encoder" <- w670
                n139 = Bundle By Name(cluster=w681, "Controls.Values.xEnc"=w672, "Controls.Values.yEnc"=w671, "Controls.Values.zEnc"=w670) -> (w680:T6)
              }
              frame #8 {
                n140 = Unbundle By Name(w693) -> ("Controls.Commands.Use software limits"=w688:bool)
                n141 = Unbundle By Name(w693) -> ("Controls.Values.xEnc"=w713:dbl, "Controls.Values.X high limit"=w712:dbl)
                n142 = Unbundle By Name(w693) -> ("Controls.Values.xEnc"=w711:dbl, "Controls.Values.X low limit"=w710:dbl)
                n143 = Unbundle By Name(w693) -> ("Controls.Values.yEnc"=w709:dbl, "Controls.Values.Y high limit"=w708:dbl)
                n144 = Unbundle By Name(w693) -> ("Controls.Values.yEnc"=w707:dbl, "Controls.Values.Y low limit"=w706:dbl)
                n145 = Unbundle By Name(w693) -> ("Controls.Values.zEnc"=w694:dbl, "Controls.Values.Z high limit"=w695:dbl)
                n146 = Unbundle By Name(w693) -> ("Controls.Values.zEnc"=w696:dbl, "Controls.Values.Z low limit"=w697:dbl)
                n147 = Greater?(x=w713, y=w712) -> (0:w705:bool)
                n148 = Greater?(x=w709, y=w708) -> (0:w703:bool)
                n149 = Less?(x=w711, y=w710) -> (x < y?=w704:bool)
                n150 = Less?(x=w707, y=w706) -> (x < y?=w699:bool)
                n151 = Greater?(x=w694, y=w695) -> (0:w687:bool)
                n152 = Less?(x=w696, y=w697) -> (x < y?=w686:bool)
                n153 = And(x=w688, y=w705) -> (x .and. y?=w701:bool)
                n154 = And(x=w688, y=w704) -> (x .and. y?=w700:bool)
                n155 = And(x=w688, y=w703) -> (x .and. y?=w692:bool)
                n156 = And(x=w688, y=w699) -> (x .and. y?=w690:bool)
                n157 = And(x=w688, y=w686) -> (x .and. y?=w691:bool)
                n158 = And(x=w688, y=w687) -> (x .and. y?=w689:bool)
                n159 = Bundle By Name(cluster=w693, "Variables.Commands.softLimit_xHigh"=w701, "Variables.Commands.softLimit_xLow"=w700, "Variables.Commands.softLimit_yHigh"=w692, "Variables.Commands.softLimit_yLow"=w690, "Variables.Commands.softLimit_zLow"=w691, "Variables.Commands.softLimit_zHigh"=w689) -> (w702:T6)
              }
              frame #9 {
                # "Get the Gamepad info"
                n160 = call-poly <vilib>:"Acquire Input Data.vi"("device ID"=w729) -> ("axis info"=w725:T9, "button info"=w720:T10)  [unwired: 1 in, 16 out]
              }
              frame #10 {
                # "Have any Gamepad buttons been pressed?"
                n161 = call "user maped buttons.vi"("previous button state"=w736, "gp button info"=w735, "map references"=w737) -> ("mapped gp buttons"=w730:T11)  [unwired: 2 out]
              }
              frame #11 {
                n162 = Unbundle By Name(w745) -> ("halt"=w746:bool)
                n163 = case shown="True" w746 {
                  selector: w746 -> [_ w751]
                  frame False {
                  }
                  frame True {
                    n164 = local write "halt 2"(w751) -> ()
                  }
                }
              }
              frame #12 {
                w760 = 0.05 ("return type")
                w792 = 0.05 ("return type")
                w793 = 0.05 ("return type")
                n165 = Unbundle("Slide 2") -> (w775:u32, w774:u32, w765:u32)
                n166 = Cluster To Array(cluster=w772) -> (array=w776:i32[])
                n167 = Index Array(array=w776, index #1=w775, index #2=w774, index #3=w765) -> (element #1=w777:i32, element #2=w773:i32, element #3=w756:i32)
                n168 = Negate(x=w756) -> (-x=w757:i32)
                n169 = Select(t=w757, s="Invert 2", f=w756) -> (s? t:f=w758:i32)
                n170 = Negate(x=w773) -> (-x=w779:i32)
                n171 = Negate(x=w777) -> (-x=w788:i32)
                n172 = Select(t=w779, s="Invert", f=w773) -> (s? t:f=w790:i32)
                n173 = Select(t=w788, s="Invert", f=w777) -> (s? t:f=w789:i32)
                n174 = Divide(x=w758, y=32768) -> (x/y=w755:dbl)
                n175 = Divide(x=w789, y=32768) -> (x/y=w781:dbl)
                n176 = Negate(x=w793) -> (-x=w794:dbl)
                n177 = Negate(x=w760) -> (-x=w761:dbl)
                n178 = Divide(x=w790, y=32768) -> (x/y=w780:dbl)
                n179 = Negate(x=w792) -> (-x=w791:dbl)
                n180 = In Range and Coerce(upper limit=w793, x=w780, lower limit=w794) -> (In Range?=w785:bool)  [unwired: 1 out]
                n181 = In Range and Coerce(upper limit=w792, x=w781, lower limit=w791) -> (In Range?=w783:bool)  [unwired: 1 out]
                n182 = In Range and Coerce(upper limit=w760, x=w755, lower limit=w761) -> (In Range?=w762:bool)  [unwired: 1 out]
                n183 = Select(t=0.0, s=w783, f=w781) -> (s? t:f=w796:dbl)
                n184 = Select(t=0.0, s=w785, f=w780) -> (s? t:f=w797:dbl)
                n185 = Select(t=0.0, s=w762, f=w755) -> (s? t:f=w764:dbl)
              }
              frame #13 {
                n186 = Unbundle By Name(w806) -> ("Controls.Values.xStep"=w809:dbl, "Controls.Values.yStep"=w808:dbl, "Controls.Values.zStep"=w805:dbl)
                n187 = call "button commands.vi"("Configuration"=w807, "Z Steps"=w805, "Motion"=w806, "Y Steps"=w808, "mapped gp buttons"=w799, "X Steps"=w809) -> ("Y distance"=w817:dbl, "Choose Button"=w802:bool, "Z distance"=w800:dbl, "X distance"=w814:dbl)  [unwired: 2 out]
                n188 = Not(x=w802) -> (.not. x?=w815:bool)
                n189 = Select(t=w813, s=w815, f=w814) -> (s? t:f=w812:dbl)
                n190 = Select(t=w817, s=w802, f=w819) -> (s? t:f=w804:dbl)
                n191 = Select(t=w800, s=w802, f=w801) -> (s? t:f=w803:dbl)
              }
              frame #14 {
                n192 = Unbundle By Name(w829) -> ("Controls.Values.xVelocity"=w831:dbl, "Controls.Values.zVelocity"=w827:dbl)
                n193 = Unbundle By Name(w829) -> ("Controls.Values.yVelocity"=w830:dbl)
                n194 = local read "Slide 2"() -> (w823:cluster{u32, u32, u32})
                n195 = local read "Slide 2"() -> (w824:cluster{u32, u32, u32})
                n196 = local read "Invert"() -> (w838:bool)
                n197 = Unbundle(w823) -> (w842:u32, w826:u32)  [unwired: 1 out]
                n198 = Unbundle(w824) -> (w841:u32)  [unwired: 2 out]
                n199 = control-ref of="halt 2"() -> (w840:refnum<vi>)
                n200 = local read "Invert"() -> (w839:bool)
                n201 = local read "Invert 2"() -> (w822:bool)
                n202 = call "move.vi"("x distance"=w821, "y distance"=w835, "z distance"=w825, "button com"=w834, "handle"=w837, "halt"=w840, "device ID"=w836, "velocityZ"=w827, "Encoder"=w832, "velocityX"=w831, "velocityY"=w830, "X Axis"=w841, "Y Axis"=w842, "Invert"=w839, "Invert 2"=w838, "Invert 3"=w822, "Z Axis"=w826) -> ()  [unwired: 2 in, 9 out]
              }
              frame #15 {
                w865 = T12 {"y reverse"=FALSE, "y foward"=FALSE, "x reverse"=FALSE, "x foward"=FALSE, "z reverse"=FALSE, "z foward"=FALSE}  # Limits
                # "Bit 3 - Y Forward Limit Switch\nBit 2 - Y Reverse Limit Switch\nBit 1 - X Forward Limit Switch\nBit 0 - X Reverse Limit Switch"
                n203 = Unbundle By Name(w867) -> ("Variables.Commands.softLimit_xLow"=w860:bool, "Variables.Commands.softLimit_xHigh"=w857:bool, "Variables.Commands.softLimit_yLow"=w854:bool, "Variables.Commands.softLimit_yHigh"=w851:bool, "Variables.Commands.softLimit_zLow"=w848:bool, "Variables.Commands.softLimit_zHigh"=w845:bool)
                n204 = dll-call lib="C:/Users/Labview/Desktop/SRR/MicroDrive_x64/Labview Examples/MicroDrive.dll" fn="MCL_MDStatus"("handle"=w871) -> ("status"=w872:u16)  [unwired: 4 in, 4 out]
                n205 = Number To Boolean Array(number=w872) -> (Boolean array=w873:bool[])
                n206 = Index Array(array=w873) -> (element #1=w874:bool, element #2=w875:bool, element #3=w876:bool, element #4=w877:bool, element #5=w863:bool, element #6=w862:bool)  [unwired: 6 in]
                n207 = Not(x=w874) -> (.not. x?=w859:bool)
                n208 = Not(x=w875) -> (.not. x?=w856:bool)
                n209 = Not(x=w876) -> (.not. x?=w853:bool)
                n210 = Not(x=w877) -> (.not. x?=w850:bool)
                n211 = Not(x=w863) -> (.not. x?=w847:bool)
                n212 = Not(x=w862) -> (.not. x?=w844:bool)
                n213 = Compound Arithmetic op=OR(w860, w859) -> (w861:bool)
                n214 = Compound Arithmetic op=OR(w857, w856) -> (w858:bool)
                n215 = Compound Arithmetic op=OR(w854, w853) -> (w855:bool)
                n216 = Compound Arithmetic op=OR(w851, w850) -> (w852:bool)
                n217 = Compound Arithmetic op=OR(w848, w847) -> (w849:bool)
                n218 = Compound Arithmetic op=OR(w845, w844) -> (w846:bool)
                n219 = Bundle By Name(cluster=w865, "x reverse"=w861, "x foward"=w858, "y reverse"=w855, "y foward"=w852, "z reverse"=w849, "z foward"=w846) -> (w864:T12)
              }
              frame #16 {
                w894 = u16 1 items=["X+", "X-", "Y+", "Y-"] ("up")
                n220 = Unbundle By Name(w889) -> ("Controls.Values.right"=w888:u16)
                n221 = Unbundle By Name(w889) -> ("Controls.Values.up"=w892:u16)
                n222 = Less Or Equal?(x=w892, y=w894) -> (x <= y?=w893:bool)
                n223 = case shown="False" w893 {
                  tunnel: w892 -> [w926 w940]
                  tunnel: w885 -> [w908 w927]
                  tunnel: [w922 w929] -> w891
                  tunnel: [w917 w928] -> w890
                  tunnel: w888 -> [w915 w932]
                  tunnel: [w907 w931] -> w887
                  tunnel: [w906 w930] -> w886
                  frame True {
                    w916 = u16 2 items=["X+", "X-", "Y+", "Y-"] ("up")
                    w925 = u16 0 items=["X+", "X-", "Y+", "Y-"] ("up")
                    n224 = Equal?(x=w926, y=w925) -> (x = y?=w918:bool)
                    n225 = Equal?(x=w915, y=w916) -> (x = y?=w909:bool)
                    n226 = Not(x=w918) -> (.not. x?=w919:bool)
                    n227 = Not(x=w909) -> (.not. x?=w914:bool)
                    n228 = Unbundle By Name(w908) -> ("x foward"=w924:bool)
                    n229 = Unbundle By Name(w908) -> ("x reverse"=w923:bool)
                    n230 = Unbundle By Name(w908) -> ("x foward"=w920:bool)
                    n231 = Unbundle By Name(w908) -> ("x reverse"=w921:bool)
                    n232 = Unbundle By Name(w908) -> ("y foward"=w910:bool)
                    n233 = Unbundle By Name(w908) -> ("y reverse"=w911:bool)
                    n234 = Unbundle By Name(w908) -> ("y foward"=w913:bool)
                    n235 = Unbundle By Name(w908) -> ("y reverse"=w912:bool)
                    n236 = Select(t=w924, s=w918, f=w923) -> (s? t:f=w922:bool)
                    n237 = Select(t=w920, s=w919, f=w921) -> (s? t:f=w917:bool)
                    n238 = Select(t=w910, s=w909, f=w911) -> (s? t:f=w907:bool)
                    n239 = Select(t=w913, s=w914, f=w912) -> (s? t:f=w906:bool)
                  }
                  frame False {
                    w939 = u16 0 items=["X+", "X-", "Y+", "Y-"] ("up")
                    w947 = u16 2 items=["X+", "X-", "Y+", "Y-"] ("up")
                    n240 = Equal?(x=w940, y=w947) -> (x = y?=w941:bool)
                    n241 = Equal?(x=w932, y=w939) -> (x = y?=w933:bool)
                    n242 = Not(x=w941) -> (.not. x?=w946:bool)
                    n243 = Not(x=w933) -> (.not. x?=w934:bool)
                    n244 = Unbundle By Name(w927) -> ("y foward"=w942:bool)
                    n245 = Unbundle By Name(w927) -> ("y reverse"=w943:bool)
                    n246 = Unbundle By Name(w927) -> ("y foward"=w945:bool)
                    n247 = Unbundle By Name(w927) -> ("y reverse"=w944:bool)
                    n248 = Unbundle By Name(w927) -> ("x foward"=w938:bool)
                    n249 = Unbundle By Name(w927) -> ("x reverse"=w937:bool)
                    n250 = Unbundle By Name(w927) -> ("x foward"=w935:bool)
                    n251 = Unbundle By Name(w927) -> ("x reverse"=w936:bool)
                    n252 = Select(t=w942, s=w941, f=w943) -> (s? t:f=w929:bool)
                    n253 = Select(t=w945, s=w946, f=w944) -> (s? t:f=w928:bool)
                    n254 = Select(t=w938, s=w933, f=w937) -> (s? t:f=w931:bool)
                    n255 = Select(t=w935, s=w934, f=w936) -> (s? t:f=w930:bool)
                  }
                }
                "left" <- w886
                "bottom" <- w890
                "right" <- w887
                "top" <- w891
                n256 = Unbundle By Name(w885) -> ("z foward"=w884:bool, "z reverse"=w882:bool)
                n257 = dll-call lib="C:/Users/Labview/Desktop/SRR/MicroDrive_x64/Labview Examples/MicroDrive.dll" fn="MCL_GetProductID"("handle"=w879) -> ("PID"=w880:u16)  [unwired: 6 in, 2 out]
                n258 = case shown="9478" w880 {
                  tunnel: w884 -> [_ w903 w905]
                  tunnel: [TRUE ("z foward") w903 w905] -> w883
                  tunnel: w882 -> [_ w902 w904]
                  tunnel: [TRUE ("z reverse") w902 w904] -> w881
                  frame Default {
                  }
                  frame 9475 {
                  }
                  frame 9478 {
                  }
                }
                "z top" <- w883
                "z bottom" <- w881
              }
              frame #17 {
                n259 = Unbundle By Name(w956) -> ("ControlRefs.Values.ROIs"=w955:refnum<vi>)
                n260 = Unbundle By Name(w956) -> ("Variables.Values.ROIs"=w954:cluster{"x":dbl, "y":dbl, "z":dbl}[])
                n261 = property class="Ring (strict)"(reference=w955) -> ("Value"=w953:u16)  [unwired: 1 in, 2 out]
                n262 = Index Array(array=w954, index=w953) -> (element=w952:cluster{"x":dbl, "y":dbl, "z":dbl})
                n263 = Unbundle By Name(w952) -> ("x"=→"M1 encoder at position":dbl, "y"=→"M2 encoder at position":dbl, "z"=→"M3 encoder at position":dbl)
              }
              frame #18 {
                n264 = Unbundle By Name(w970) -> ("ControlRefs.Commands.roiMoveTo"=w968:refnum<vi>, "Variables.Values.roiNumItems"=w965:i32, "ControlRefs.Commands.rename"=w963:refnum<vi>)
                n265 = Equal To 0?(x=w965) -> (x = 0?=w969:bool)
                n266 = Select(t=u8 2 ("Disabled"), s=w969, f=u8 0 ("Disabled")) -> (s? t:f=w962:u8)
                n267 = property class="Bool"(reference=w968, "Disabled"=w962) -> ()  [unwired: 1 in, 2 out]
                n268 = property class="Bool"(reference=w963, "Disabled"=w962) -> ()  [unwired: 1 in, 2 out]
              }
              frame #19 {
                n269 = Unbundle By Name(w982) -> ("Controls.Commands.roiAdd"=w983:bool)
                n270 = Unbundle By Name(w978) -> ("Controls.Values.xEnc"=w981:dbl, "Controls.Values.yEnc"=w980:dbl)
                n271 = case shown="True" w983 {
                  tunnel: w982 -> [w987 w992]
                  tunnel: w981 -> [_ _]
                  tunnel: w980 -> [_ _]
                  tunnel: [w987 w1012] -> w979
                  tunnel: w978 -> [_ w1006]
                  frame False {
                  }
                  frame True {
                    w989 = ""  # f
                    n272 = Unbundle By Name(w992) -> ("Variables.Values.roiNumItems"=w997:i32)
                    n273 = Unbundle By Name(w992) -> ("ControlRefs.Values.ROIs"=w999:refnum<vi>)
                    n274 = Increment(x=w997) -> (x+1=w991:i32)
                    n275 = Number To Decimal String(number=w991) -> (decimal integer string=w995:string)  [unwired: 1 out]
                    n276 = Unbundle By Name(w992) -> ("Variables.Values.roiText"=w994:string[])
                    n277 = Concatenate Strings("Pos" ("string"), w995) -> (w1000:string)
                    n278 = Empty String/Path?(string/path="") -> (empty?=w1001:bool)
                    n279 = Select(t=w1000, s=w1001, f=w989) -> (s? t:f=w993:string)
                    n280 = Build Array (concatenate)(w994, w993) -> (w998:string[])
                    n281 = Unbundle By Name(w1006) -> ("Controls.Values.xEnc"=w1005:dbl, "Controls.Values.yEnc"=w1003:dbl, "Controls.Values.zEnc"=w988:dbl)
                    n282 = Unbundle By Name(w992) -> ("Variables.Values.ROIs"=w1007:cluster{"x":dbl, "y":dbl, "z":dbl}[])
                    n283 = property class="Ring (strict)"(reference=w999, "Strings []"=w998) -> (reference out=w1011:refnum<vi>)  [unwired: 1 in, 1 out]
                    n284 = property class="Ring (strict)"(reference=w1011) -> (reference out=w1010:refnum<vi>, "NumItems"=w1009:u32)  [unwired: 1 in, 1 out]
                    n285 = Bundle("xEnc"=w1005, "yEnc"=w1003, "zEnc"=w988) -> (w1004:cluster{"xEnc":dbl, "yEnc":dbl, "zEnc":dbl})  [unwired: 1 out]
                    n286 = Build Array (concatenate)(w1007, w1004) -> (w1002:cluster{"xEnc":dbl, "yEnc":dbl, "zEnc":dbl}[])
                    n287 = Bundle By Name(cluster=w992, "Variables.Values.roiText"=w998, "Variables.Values.ROIs"=w1002, "Variables.Values.roiNumItems"=w991) -> (w1012:T7)
                    n288 = Decrement(x=w1009) -> (x-1=w1008:u32)
                    n289 = property class="Ring (strict)"(reference=w1010, "Value"=w1008) -> ()  [unwired: 1 in, 2 out]
                  }
                }
              }
              frame #20 {
                n290 = Unbundle By Name(w1021) -> ("Variables.Values.roiText"=w1018:string[], "ControlRefs.Values.ROIs"=w1019:refnum<vi>, "Controls.Commands.rename"=w1022:bool, "Controls.Values.roiName"=w1015:string, "ControlRefs.Values.ROIs"=w1017:refnum<vi>)
                n291 = Empty String/Path?(string/path=w1015) -> (empty?=w1014:bool)
                n292 = Not(x=w1014) -> (.not. x?=w1013:bool)
                n293 = Compound Arithmetic op=AND(w1022, w1013) -> (w1016:bool)
                n294 = case shown="True" w1016 {
                  tunnel: [w1029 w1037] -> w1020
                  tunnel: w1021 -> [w1029 w1036]
                  tunnel: w1019 -> [_ w1035]
                  tunnel: w1018 -> [_ w1034]
                  tunnel: w1015 -> [_ w1032]
                  tunnel: w1017 -> [_ w1031]
                  frame False {
                  }
                  frame True {
                    n295 = property class="Ring (strict)"(reference=w1035) -> ("Value"=w1033:u16)  [unwired: 1 in, 2 out]
                    n296 = Replace Array Subset(array=w1034, new element=w1032, index=w1033) -> (w1030:string[])
                    n297 = Bundle By Name(cluster=w1036, "Variables.Values.roiText"=w1030) -> (w1037:T7)
                    n298 = property class="Ring (strict)"(reference=w1031, "Strings []"=w1030) -> ()  [unwired: 1 in, 2 out]
                  }
                }
              }
              frame #21 {
                n299 = Unbundle By Name(w1046) -> ("Controls.Commands.roiDelete"=w1040:bool, "Variables.Values.roiNumItems"=w1041:i32)
                n300 = Greater Than 0?(x=w1041) -> (x > 0?=w1039:bool)
                n301 = Compound Arithmetic op=AND(w1040, w1039) -> (w1038:bool)
                n302 = case shown="True" w1038 {
                  tunnel: w1046 -> [w1050 w1058]
                  tunnel: [w1050 w1063] -> w1044
                  tunnel: w1045 -> [_ _]
                  frame False {
                  }
                  frame True {
                    n303 = Unbundle By Name(w1058) -> ("Variables.Values.ROIs"=w1055:cluster{"x":dbl, "y":dbl, "z":dbl}[], "Variables.Values.roiNumItems"=w1052:i32)
                    n304 = Unbundle By Name(w1058) -> ("ControlRefs.Values.ROIs"=w1064:refnum<vi>, "Variables.Values.roiText"=w1057:string[], "Controls.Values.ROIs"=w1054:u16)
                    n305 = Decrement(x=w1052) -> (x-1=w1051:i32)
                    n306 = Delete From Array(array=w1057, index=w1054) -> (array with subset deleted=w1056:string[])  [unwired: 1 in, 1 out]
                    n307 = Delete From Array(array=w1055, index=w1054) -> (array with subset deleted=w1053:cluster{"x":dbl, "y":dbl, "z":dbl}[])  [unwired: 1 in, 1 out]
                    n308 = property class="Ring (strict)"(reference=w1064, "Strings []"=w1056) -> (reference out=w1062:refnum<vi>)  [unwired: 1 in, 1 out]
                    n309 = Bundle By Name(cluster=w1058, "Variables.Values.roiText"=w1056, "Variables.Values.ROIs"=w1053, "Variables.Values.roiNumItems"=w1051) -> (w1063:T7)
                    n310 = property class="Ring (strict)"(reference=w1062) -> (reference out=w1061:refnum<vi>, "NumItems"=w1060:u32)  [unwired: 1 in, 1 out]
                    n311 = Decrement(x=w1060) -> (x-1=w1059:u32)
                    n312 = property class="Ring (strict)"(reference=w1061, "Value"=w1059) -> ()  [unwired: 1 in, 2 out]
                  }
                }
              }
              frame #22 {
                n313 = Unbundle By Name(w1068) -> ("Controls.Commands.roiDeleteAll"=w1069:bool)
                n314 = case shown="True" w1069 {
                  tunnel: w1068 -> [w1074 w1080]
                  tunnel: [w1074 w1081] -> w1066
                  tunnel: w1067 -> [_ _]
                  frame False {
                  }
                  frame True {
                    w1077 = string[] [] ("Strings []")
                    w1079 = u16 0  # Value
                    n315 = Unbundle By Name(w1080) -> ("ControlRefs.Values.ROIs"=w1082:refnum<vi>)
                    n316 = Bundle By Name(cluster=w1080, "Variables.Values.roiText"=w1077, "Variables.Values.ROIs"=cluster{"x":dbl, "y":dbl, "z":dbl}[] [], "Variables.Values.roiNumItems"=0) -> (w1081:T7)
                    n317 = property class="Ring (strict)"(reference=w1082, "Strings []"=w1077) -> (reference out=w1078:refnum<vi>)  [unwired: 1 in, 1 out]
                    n318 = property class="Ring (strict)"(reference=w1078, "Value"=w1079) -> ()  [unwired: 1 in, 2 out]
                  }
                }
              }
              frame #23 {
                n319 = Unbundle By Name(w1088) -> ("Controls.Commands.roiMoveTo"=w1089:bool)
                n320 = case shown="True" w1089 {
                  tunnel: w1088 -> [_ w1118]
                  tunnel: w1087 -> [_ w1117]
                  tunnel: w1086 -> [_ w1116]
                  tunnel: w1085 -> [_ w1115]
                  tunnel: w1084 -> [_ w1114]
                  frame False {
                  }
                  frame True {
                    w1101 = u16 4 items=["X axis", "Y axis", "Z axis", "X axis rotation", "Y axis rotation", "Z axis rotation", "U axis", "V axis"] ("Y Axis")
                    w1105 = u16 0 items=["X axis", "Y axis", "Z axis", "X axis rotation", "Y axis rotation", "Z axis rotation", "U axis", "V axis"] ("Y Axis")
                    w1106 = u16 1 items=["X axis", "Y axis", "Z axis", "X axis rotation", "Y axis rotation", "Z axis rotation", "U axis", "V axis"] ("Y Axis")
                    w1107 = FALSE  # Invert
                    w1108 = FALSE  # Invert 2
                    w1111 = TRUE  # button com
                    n321 = Unbundle By Name(w1118) -> ("Variables.Values.ROIs"=w1092:cluster{"x":dbl, "y":dbl, "z":dbl}[], "Controls.Values.ROIs"=w1091:u16)
                    n322 = Index Array(array=w1092, index=w1091) -> (element=w1093:cluster{"x":dbl, "y":dbl, "z":dbl})
                    n323 = Unbundle By Name(w1117) -> ("Controls.Values.yEnc"=w1096:dbl)
                    n324 = Unbundle By Name(w1117) -> ("Controls.Values.xEnc"=w1098:dbl)
                    n325 = Unbundle By Name(w1117) -> ("Controls.Values.zEnc"=w1095:dbl)
                    n326 = Unbundle By Name(w1093) -> ("x"=w1099:dbl)
                    n327 = Unbundle By Name(w1093) -> ("y"=w1097:dbl)
                    n328 = Unbundle By Name(w1093) -> ("z"=w1094:dbl)
                    n329 = Subtract(x=w1099, y=w1098) -> (x-y=w1102:dbl)
                    n330 = Subtract(x=w1097, y=w1096) -> (x-y=w1112:dbl)
                    n331 = Subtract(x=w1094, y=w1095) -> (x-y=w1100:dbl)
                    n332 = Unbundle By Name(w1116) -> ("Controls.Values.xVelocity"=w1110:dbl, "Controls.Values.zVelocity"=w1104:dbl)
                    n333 = Unbundle By Name(w1116) -> ("Controls.Values.yVelocity"=w1109:dbl)
                    n334 = control-ref of="halt 2"() -> (w1113:refnum<vi>)
                    n335 = call "move.vi"("x distance"=w1102, "y distance"=w1112, "z distance"=w1100, "button com"=w1111, "handle"=w1115, "halt"=w1113, "device ID"=w1114, "velocityZ"=w1104, "Encoder"=w1117, "velocityX"=w1110, "velocityY"=w1109, "X Axis"=w1105, "Y Axis"=w1106, "Invert"=w1107, "Invert 2"=w1108, "Invert 3"=FALSE, "Z Axis"=w1101) -> ()  [unwired: 2 in, 9 out]
                  }
                }
              }
              frame #24 {
                n336 = Unbundle By Name(w1119) -> ("Controls.Commands.roiSave"=w1122:bool)
                n337 = Unbundle By Name(w1119) -> ("Variables.Values.roiText"=w1121:string[], "Variables.Values.ROIs"=w1120:cluster{"x":dbl, "y":dbl, "z":dbl}[])
                n338 = case shown="True" w1122 {
                  tunnel: w1121 -> [_ w1131]
                  tunnel: w1120 -> [_ w1130]
                  frame False {
                  }
                  frame True {
                    n339 = flat-sequence {
                      tunnel: w1131 -> [w1134]
                      tunnel: w1130 -> [w1133]
                      tunnel: [w1132] -> w1129
                      tunnel: w1129 -> [w1163]
                      frame #0 {
                        n340 = for {
                          tunnel: w1134 -> [w1143] mode=indexing
                          tunnel: w1133 -> [w1146] mode=indexing
                          tunnel: [w1138] -> w1132 mode=indexing
                          n341 = Unbundle By Name(w1146) -> ("x"=w1144:dbl, "y"=w1145:dbl, "z"=w1137:dbl)
                          n342 = Number To Fractional String(number=w1137) -> (F-format string=w1136:string)  [unwired: 3 out]
                          n343 = Number To Fractional String(number=w1145) -> (F-format string=w1139:string)  [unwired: 3 out]
                          n344 = Number To Fractional String(number=w1144) -> (F-format string=w1141:string)  [unwired: 3 out]
                          n345 = Concatenate Strings(w1143, "\t", w1141, "\t", w1139, "\t", w1136) -> (w1138:string)
                        }
                      }
                      frame #1 {
                        n346 = Delete From Array(array=w1163, index=0) -> (deleted portion=w1161:string, array with subset deleted=w1160:string[])  [unwired: 1 in]
                        n347 = Get Date/Time String() -> (date string=w1157:string, time string=w1148:string)  [unwired: 3 out]
                        n348 = call <vilib>:"Space Constant.vi"() -> ("String"=w1149:string)
                        n349 = for {
                          tunnel: w1160 -> [w1170] mode=indexing
                          shift-right: [w1171] -> w1164
                          shift-left: w1161 -> [w1172]
                          n350 = Concatenate Strings(w1172, "\r\n", w1170) -> (w1171:string)
                        }
                        n351 = Concatenate Strings(w1157, w1149, w1148) -> (w1156:string)
                        n352 = Search and Replace String(replace all?=TRUE ("replace all? (F)"), input string=w1156, search string=":") -> (result string=w1154:string)  [unwired: 1 in, 7 out]
                        n353 = Search and Replace String(replace all?=TRUE ("replace all? (F)"), input string=w1154, search string="/", replace string="-" ("replace string (\"\")")) -> (result string=w1158:string)  [unwired: 1 in, 6 out]
                        n354 = Concatenate Strings("positions " ("string"), w1158) -> (w1147:string)
                        n355 = call "File Dialog"("default name"=w1147, "pattern (all files)"="*.txt") -> ("selected path"=w1166:path, "cancelled"=w1167:bool, "error out"=w1165:errorcluster)  [unwired: 5 in, 6 out]
                        n356 = case shown="False" w1167 {
                          tunnel: w1166 -> [w1174 _]
                          tunnel: w1165 -> [_ _]
                          tunnel: w1164 -> [w1173 _]
                          frame False {
                            n357 = Write to Text File(file (use dialog)=w1174, text=w1173) -> ()  [unwired: 1 in, 4 out]
                          }
                          frame True {
                          }
                        }
                      }
                    }
                  }
                }
              }
              frame #25 {
                n358 = Unbundle By Name(w1176) -> ("Controls.Commands.roiLoad"=w1177:bool)
                n359 = case shown="True" w1177 {
                  tunnel: w1176 -> [w1184 w1186]
                  tunnel: [w1184 w1185] -> w1175
                  frame False {
                  }
                  frame True {
                    n360 = flat-sequence {
                      tunnel: w1186 -> [w1188]
                      tunnel: [w1187] -> w1185
                      frame #0 {
                        n361 = call "File Dialog2"("pattern (all files)"="*.txt") -> ("selected path"=w1191:path, "cancelled"=w1190:bool, "error out"=w1192:errorcluster)  [unwired: 6 in, 6 out]
                        n362 = case shown="False" w1190 {
                          tunnel: w1191 -> [w1204 _]
                          tunnel: w1192 -> [_ _]
                          tunnel: w1188 -> [w1197 w1250]
                          tunnel: [w1193 w1250] -> w1187
                          frame False {
                            n363 = flat-sequence {
                              tunnel: w1204 -> [w1207]
                              tunnel: [w1206] -> w1203
                              tunnel: w1197 -> [w1205]
                              tunnel: [w1205] -> w1195
                              tunnel: w1203 -> [w1213]
                              tunnel: [w1213] -> w1202
                              tunnel: [w1209] -> w1201
                              tunnel: [w1208] -> w1196
                              tunnel: w1195 -> [w1208]
                              tunnel: w1202 -> [w1222]
                              tunnel: w1201 -> [w1221]
                              tunnel: [w1222] -> w1200
                              tunnel: [w1220] -> w1199
                              tunnel: [w1219] -> w1198
                              tunnel: w1196 -> [w1218]
                              tunnel: [w1218] -> w1194
                              tunnel: [w1249] -> _
                              tunnel: w1200 -> [w1249]
                              tunnel: w1199 -> [w1248]
                              tunnel: w1198 -> [w1243]
                              tunnel: w1194 -> [w1246]
                              tunnel: [w1247] -> w1193
                              frame #0 {
                                n364 = Read from Text File(file (use dialog)=w1207) -> (text=w1206:string)  [unwired: 1 in, 5 out]
                              }
                              frame #1 {
                                n365 = while {
                                tunnel: w1213 -> [w1216]
                                tunnel: [w1214] -> w1212 mode=indexing
                                i -> [w1217]
                                stop <- w1215 stop-if-true
                                n366 = Pick Line(multi-line string=w1216, line index=w1217) -> (output string=w1214:string)  [unwired: 1 out]
                                n367 = Empty String/Path?(string/path=w1214) -> (empty?=w1215:bool)
                                }
                                n368 = Array Size(array=w1212) -> (size(s)=w1211:i32)
                                n369 = Decrement(x=w1211) -> (x-1=w1210:i32)
                                n370 = Delete From Array(array=w1212, index=w1210) -> (array with subset deleted=w1209:string[])  [unwired: 1 in, 1 out]
                              }
                              frame #2 {
                                n371 = for {
                                tunnel: w1221 -> [w1242] mode=indexing
                                tunnel: [w1235] -> w1220 mode=indexing
                                tunnel: [w1234] -> w1219 mode=indexing
                                w1238 = cluster{"x":dbl, "y":dbl, "z":dbl} {"x"=0.0, "y"=0.0, "z"=0.0}  # ROI
                                n372 = Search/Split String(string=w1242, search string/char (-)="\t") -> (substring before match=w1234:string, match + rest of string=w1239:string)  [unwired: 2 out]
                                n373 = Search/Split String(string=w1239, search string/char (-)="\t", offset (0)=1) -> (substring before match=w1237:string, match + rest of string=w1227:string)  [unwired: 1 out]
                                n374 = Search/Split String(string=w1227, search string/char (-)="\t", offset (0)=1) -> (substring before match=w1226:string, match + rest of string=w1225:string)  [unwired: 1 out]
                                n375 = Fract/Exp String To Number(string=w1225, offset=1) -> (number=w1228:dbl)  [unwired: 3 out]
                                n376 = Fract/Exp String To Number(string=w1226, offset=1) -> (number=w1230:dbl)  [unwired: 3 out]
                                n377 = Fract/Exp String To Number(string=w1237, offset=1) -> (number=w1236:dbl)  [unwired: 3 out]
                                n378 = Bundle By Name(cluster=w1238, "x"=w1236, "y"=w1230, "z"=w1228) -> (w1235:cluster{"x":dbl, "y":dbl, "z":dbl})
                                }
                              }
                              frame #3 {
                                n379 = Array Size(array=w1243) -> (size(s)=w1244:i32)
                                n380 = Unbundle By Name(w1246) -> ("ControlRefs.Values.ROIs"=w1245:refnum<vi>)
                                n381 = Bundle By Name(cluster=w1246, "Variables.Values.roiNumItems"=w1244, "Variables.Values.roiText"=w1243, "Variables.Values.ROIs"=w1248) -> (w1247:T7)
                                n382 = property class="Ring (strict)"(reference=w1245, "Strings []"=w1243) -> ()  [unwired: 1 in, 2 out]
                              }
                            }
                          }
                          frame True {
                          }
                        }
                      }
                    }
                  }
                }
              }
              frame #26 {
                n383 = Unbundle By Name(w1258) -> ("Controls.Commands.saveLimits"=w1257:bool, "Controls.Values.X high limit"=w1256:dbl, "Controls.Values.X low limit"=w1255:dbl, "Controls.Values.Y high limit"=w1254:dbl, "Controls.Values.Y low limit"=w1253:dbl, "Controls.Values.Z high limit"=w1252:dbl, "Controls.Values.Z low limit"=w1251:dbl)
                n384 = case shown="True" w1257 {
                  tunnel: w1256 -> [_ w1270]
                  tunnel: w1255 -> [_ w1269]
                  tunnel: w1254 -> [_ w1268]
                  tunnel: w1253 -> [_ w1267]
                  tunnel: w1252 -> [_ w1266]
                  tunnel: w1251 -> [_ w1265]
                  frame False {
                  }
                  frame True {
                    n385 = flat-sequence {
                      tunnel: w1267 -> [w1286]
                      tunnel: w1268 -> [w1287]
                      tunnel: w1269 -> [w1288]
                      tunnel: w1270 -> [w1289]
                      tunnel: w1266 -> [w1272]
                      tunnel: w1265 -> [w1271]
                      frame #0 {
                        n386 = Get Date/Time String() -> (date string=w1276:string, time string=w1285:string)  [unwired: 3 out]
                        n387 = call <vilib>:"Space Constant.vi"() -> ("String"=w1284:string)
                        n388 = Build Array(w1289, w1288, w1287, w1286, w1272, w1271) -> (w1290:dbl[])
                        n389 = Concatenate Strings(w1276, w1284, w1285) -> (w1277:string)
                        n390 = Search and Replace String(replace all?=TRUE ("replace all? (F)"), input string=w1277, search string=":") -> (result string=w1279:string)  [unwired: 1 in, 7 out]
                        n391 = Search and Replace String(replace all?=TRUE ("replace all? (F)"), input string=w1279, search string="/", replace string="-" ("replace string (\"\")")) -> (result string=w1275:string)  [unwired: 1 in, 6 out]
                        n392 = Concatenate Strings("limits " ("string"), w1275) -> (w1274:string)
                        n393 = call "File Dialog3"("default name"=w1274, "pattern (all files)"="*.txt") -> ("selected path"=w1292:path, "cancelled"=w1293:bool, "error out"=w1291:errorcluster)  [unwired: 5 in, 6 out]
                        n394 = case shown="False" w1293 {
                          tunnel: w1292 -> [w1295 _]
                          tunnel: w1291 -> [_ _]
                          tunnel: w1290 -> [w1298 _]
                          frame False {
                            n395 = call-poly <vilib>:"Write To Spreadsheet File.vi"("transpose? (no:F)"=TRUE, "format (%.3f)"="%.6f", "1D data"=w1298, "file path (dialog if empty)"=w1295) -> ()  [unwired: 2 in, 3 out]
                          }
                          frame True {
                          }
                        }
                      }
                    }
                  }
                }
              }
              frame #27 {
                n396 = Unbundle By Name(w1299) -> ("Controls.Commands.loadLimits"=w1300:bool)
                n397 = case shown="True" w1300 {
                  tunnel: w1299 -> [_ w1307]
                  frame False {
                  }
                  frame True {
                    n398 = flat-sequence {
                      tunnel: w1307 -> [w1308]
                      frame #0 {
                        n399 = call "File Dialog4"("pattern (all files)"="*.txt") -> ("selected path"=w1310:path, "cancelled"=w1311:bool, "error out"=w1309:errorcluster)  [unwired: 6 in, 6 out]
                        n400 = case shown="False" w1311 {
                          tunnel: w1310 -> [w1326 _]
                          tunnel: w1309 -> [_ _]
                          tunnel: w1308 -> [w1327 _]
                          frame False {
                            n401 = Unbundle By Name(w1327) -> ("ControlRefs.Values.X high limit"=w1325:refnum<vi>, "ControlRefs.Values.X low limit"=w1324:refnum<vi>, "ControlRefs.Values.Y high limit"=w1323:refnum<vi>, "ControlRefs.Values.Y low limit"=w1322:refnum<vi>, "ControlRefs.Values.Z high limit"=w1314:refnum<vi>, "ControlRefs.Values.Z low limit"=w1313:refnum<vi>)
                            n402 = call-poly <vilib>:"Read From Spreadsheet File.vi"("transpose (no:F)"=TRUE ("transpose? (no:F)"), "format (%.3f)"="%.6f", "file path (dialog if empty)"=w1326) -> ("first row"=w1321:dbl[])  [unwired: 1 in, 7 out]
                            n403 = Index Array(array=w1321) -> (element #1=w1320:dbl, element #2=w1319:dbl, element #3=w1318:dbl, element #4=w1317:dbl, element #5=w1316:dbl, element #6=w1315:dbl)  [unwired: 6 in]
                            n404 = property class="DigNum (strict)"(reference=w1325, "Value"=w1320) -> ()  [unwired: 1 in, 2 out]
                            n405 = property class="DigNum (strict)"(reference=w1324, "Value"=w1319) -> ()  [unwired: 1 in, 2 out]
                            n406 = property class="DigNum (strict)"(reference=w1323, "Value"=w1318) -> ()  [unwired: 1 in, 2 out]
                            n407 = property class="DigNum (strict)"(reference=w1322, "Value"=w1317) -> ()  [unwired: 1 in, 2 out]
                            n408 = property class="DigNum (strict)"(reference=w1314, "Value"=w1316) -> ()  [unwired: 1 in, 2 out]
                            n409 = property class="DigNum (strict)"(reference=w1313, "Value"=w1315) -> ()  [unwired: 1 in, 2 out]
                          }
                          frame True {
                          }
                        }
                      }
                    }
                  }
                }
              }
              frame #28 {
              }
            }
          }
          n410 = dll-call lib="C:/Users/Labview/Desktop/SRR/MicroDrive_x64/Labview Examples/MicroDrive.dll" fn="MCL_ReleaseHandle"("handle"=w291) -> ()  [unwired: 4 in, 3 out]
          n411 = call-poly <vilib>:"Close Input Device.vi"("device ID"=w292) -> ()  [unwired: 1 in, 9 out]
          n412 = event shown="[1] Panel Close?" {
            selector: _ -> [_ _]
            dyn-events: _ -> [_ _]
            timeout: -1 -> [_ _]
            event Timeout {
              n413 = event-data() -> ()  [unwired: 3 out]
            }
            event Panel Close? {
              n414 = event-data() -> ()  [unwired: 4 out]
              n415 = local write "closed?"(TRUE ("closed?")) -> ()
              n416 = event-data("Discard?"=TRUE) -> ()  [unwired: 1 in, 1 out]
            }
          }
        }
      }
    }
  }
